vi "art联动采集V4.9(新增双行扫描模块).vi"() -> ()   [LabVIEW 2016]
uses:
  <vilib>/Utility/file.llb/Read Delimited Spreadsheet (I64).vi
  <vilib>/Instr/_visa.llb/VISA Configure Serial Port (Instr).vi
  <vilib>/Utility/file.llb/Write Delimited Spreadsheet (DBL).vi
panel:
  in  "单行？":enum32{"单行", "双行"}(radio)
  in  "色码表导入":path=path "C:/Users/H301/Desktop/art闭环扫描程序/色码表/色码表（黑白）.txt" caption="（色码表导入）"
  out "水平进度条":u8(slide) scale=0.0..100.0
  out "x+y 3":dbl=3.0
  in  "分层图查看":bool
  in  "hDevice 2":i32
  in  "逐行扫描":bool
  in  "定位模式":bool
  in  "X终点":dbl
  in  "Y终点":dbl
  in  "高级设置":bool
  in  "Y轴回零速度":dbl=15000.0
  in  "X轴回零速度":dbl=15000.0
  in  "细分设置":dbl=8.0
  in  "等待时间":u32=40
  in  "文件保存":path=path "C:/Users/H301/Desktop/art采集实验数据" caption="保存路径"
  out "已用时（s）":dbl format="%<%H:%M:%S>t"
  out "error out":errorcluster caption="错误输出"
  in  "退出扫描(Esc)":bool
  in  "N_Length":i32=1048576
  out "M_Length":i32
  out "hDevice":i32=241832032
  out "pulDDR2Length":u32=256
  out "毫秒计时值":u32=3586537
  out "数组":dbl[][](array[numeric])=[[58819.77200735986, 88200.32943600747]]
  out "强度图":dbl[][](graph)=[[58819.77200735986, 88200.32943600747]]
  out "judge":dbl
  out "Xloop":dbl
  out "幅频谱":dbl[](graph)
  out "时域谱":dbl[](graph)
  out "错误输出":errorcluster
  in  "启动":bool
  in  "逐点扫描":bool
  in  "X归零":bool
  in  "Y归零":bool
  in  "Y起点":dbl
  in  "Y轴速度":dbl=9000.0
  in  "X轴速度":dbl=9000.0
  out "电机状态":bool
  in  "电机端口":refnum<visa-resource-name>="COM6"
  out "Yloop":dbl=1.0
  out "X扫描范围":dbl=150.0
  out "Y扫描范围":dbl=75.0
  out "Y序":i32
  in  "X起点":dbl
  out "Y(mm)":dbl
  out "x+y 2":dbl=3.0
  in  "Y:":dbl=1.0
  in  "精度":dbl=0.001
  in  "电机急停":bool
  out "X（mm）":dbl
  out "x+y":dbl=1.0
  in  "X:":dbl=1.0
  # "实时坐标"
  # "时域谱"
  # "频域谱"
  # "归零"
  # "扫描区域"
  # "扫描步进(mm)"
  # "X:"
  # "~"
  # "Y:"
  # "~"
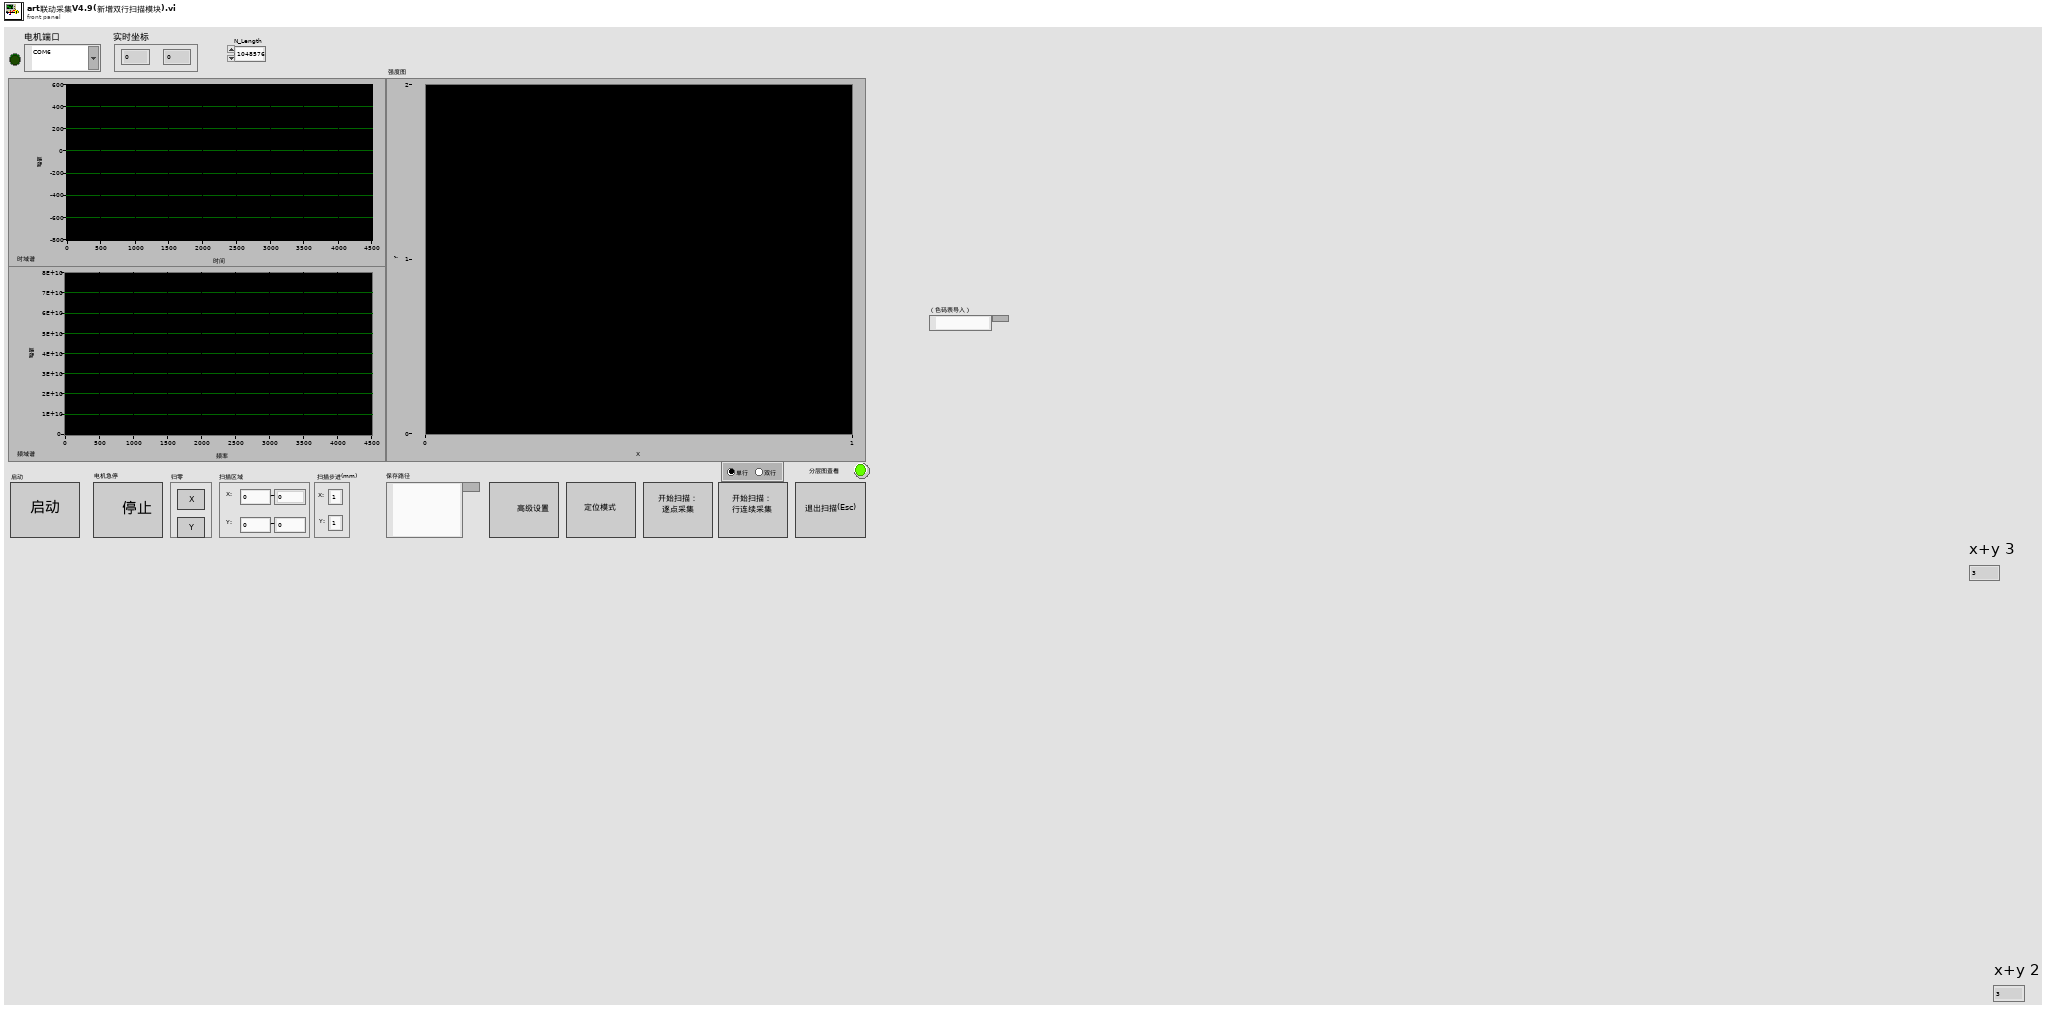
[diagram p1: front panel]
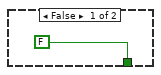
[diagram p2: hidden frame]
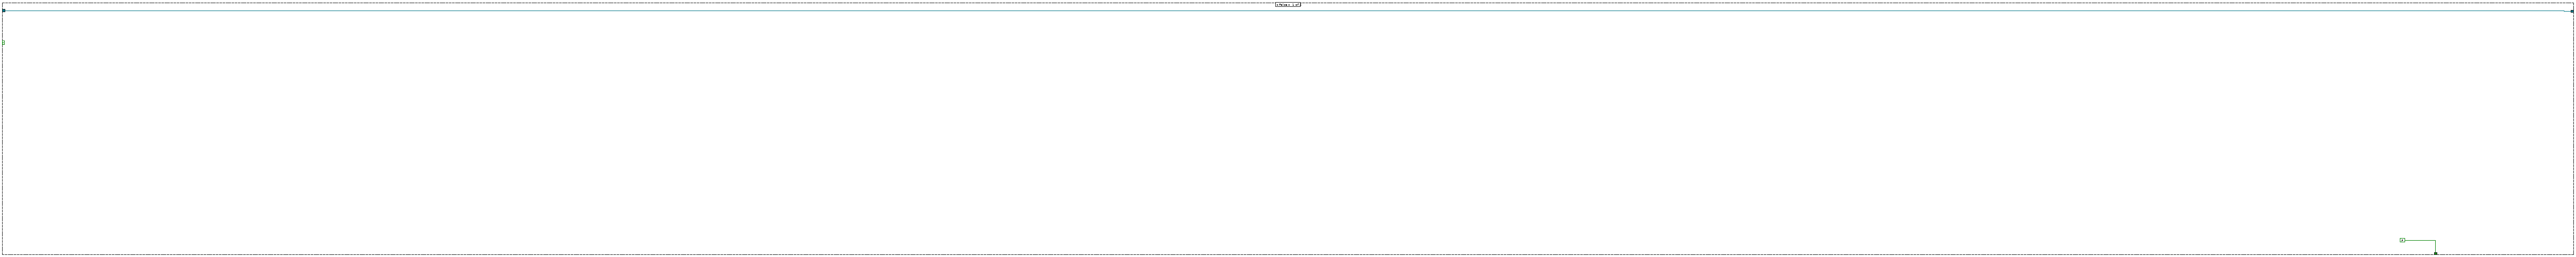
[diagram p3: hidden frame]
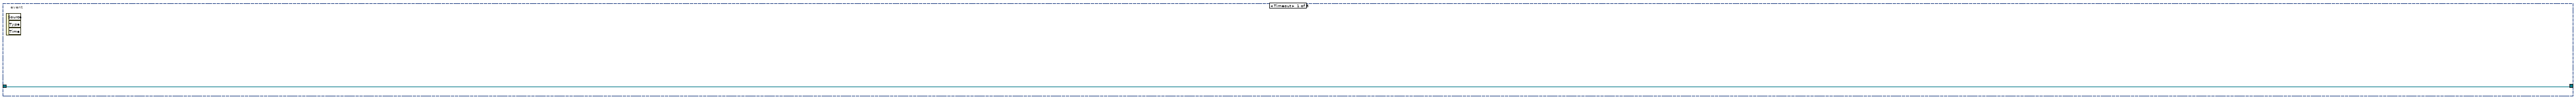
[diagram p4: hidden frame]
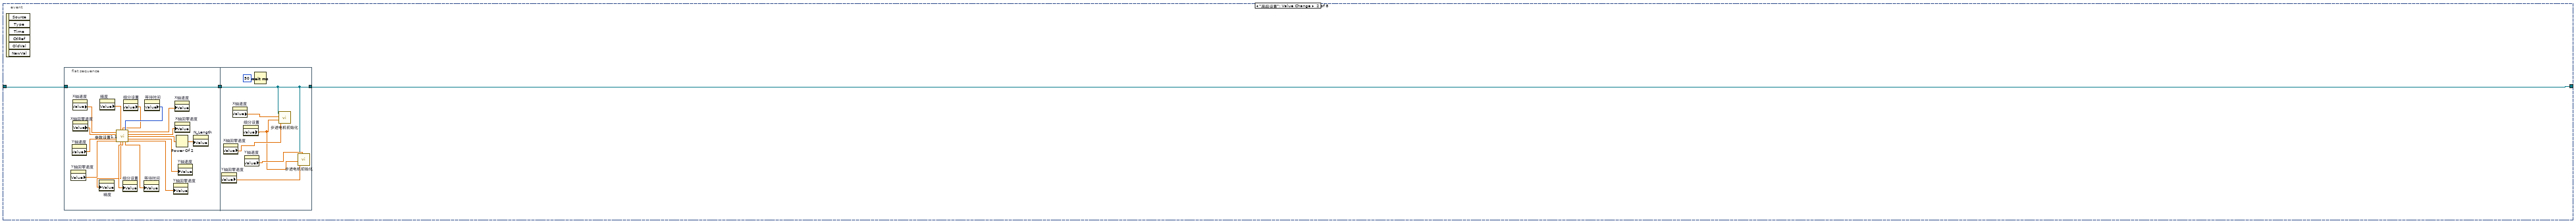
[diagram p5: hidden frame]
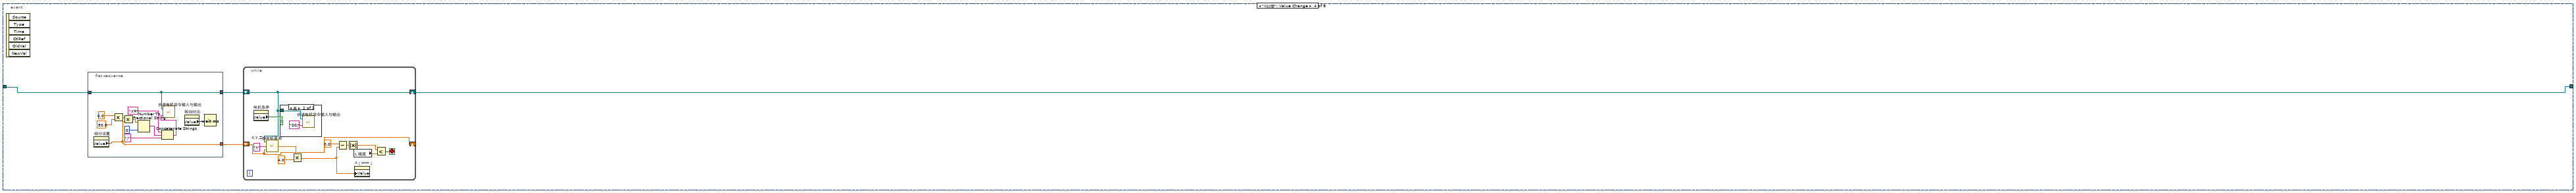
[diagram p6: hidden frame]
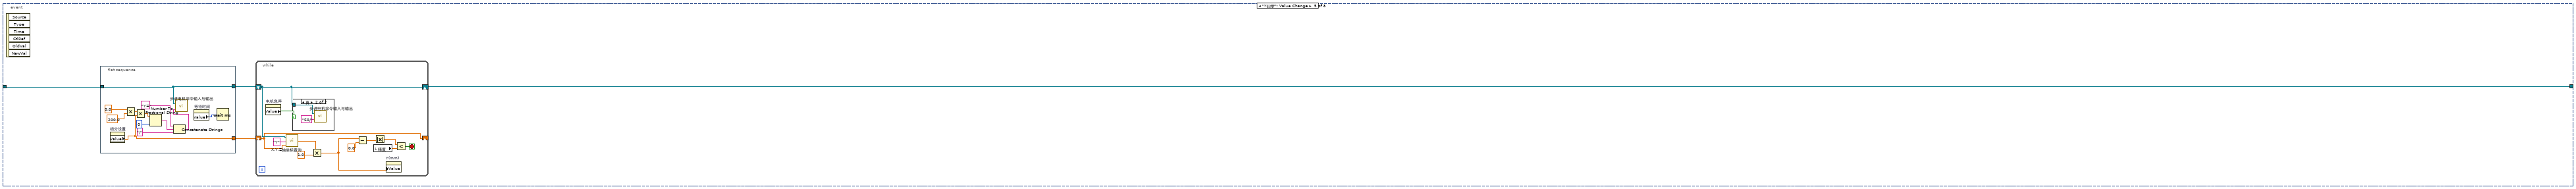
[diagram p8: hidden frame]
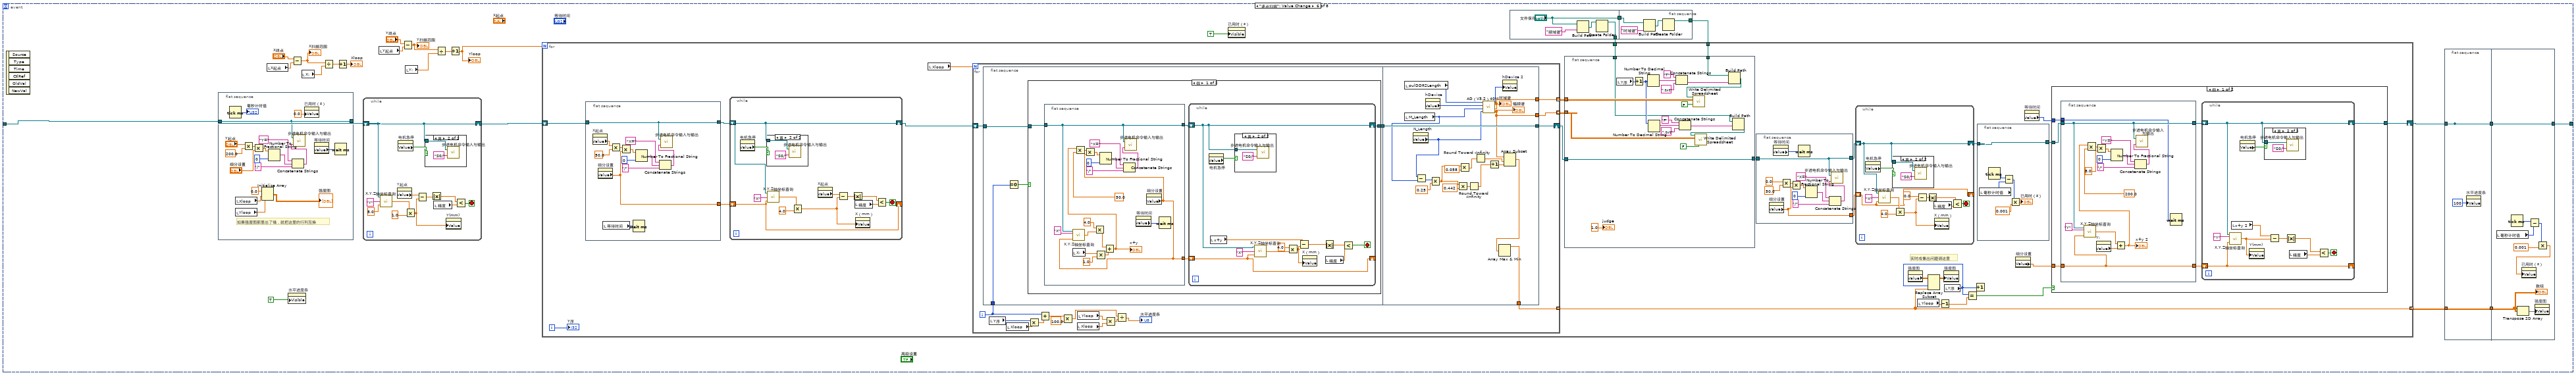
[diagram p10: hidden frame]
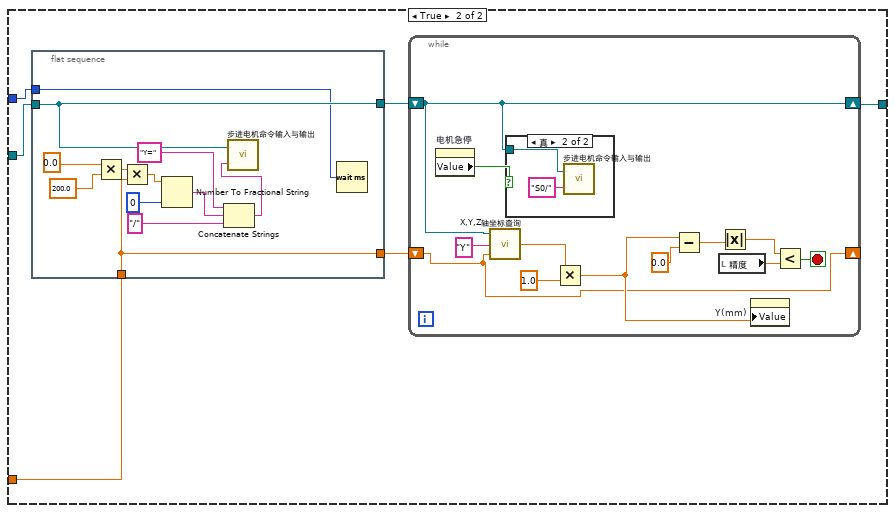
[diagram p15: hidden frame]
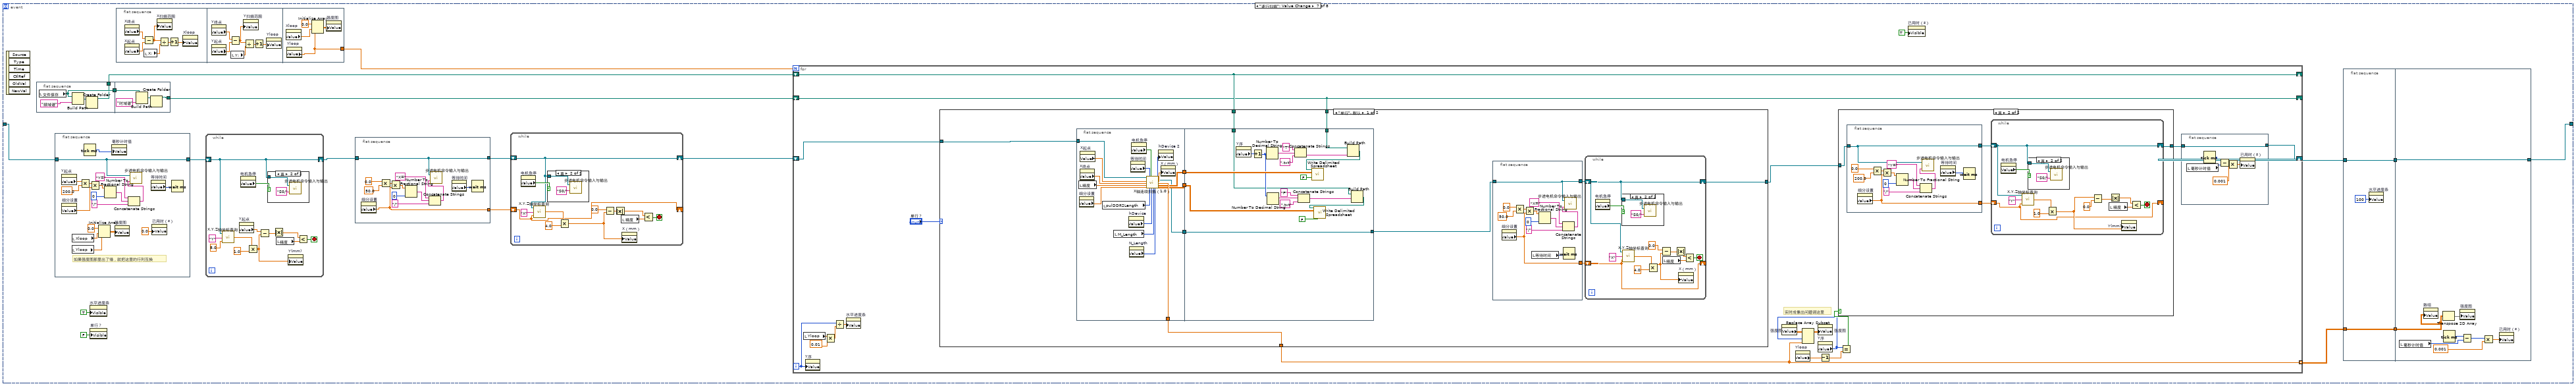
[diagram p19: hidden frame]
diagram:
  n1 = call-poly <vilib>:"Read Delimited Spreadsheet.vi"("file path (dialog if empty)"="色码表导入") -> ("first row"=w2:i64[])  [unwired: 9 in, 5 out]
  n2 = property on="强度图" class="IntGraph (严格)"("Color Table"=w2) -> ()  [unwired: 2 in, 2 out]
  n3 = property on="水平进度条" class="Slide (严格)"("Visible"=FALSE ("可见")) -> ()  [unwired: 2 in, 2 out]
  n4 = property on="单行？" class="RadioBtnsControl (严格)"("Visible"=TRUE ("可见")) -> ()  [unwired: 2 in, 2 out]
  n5 = while {
    stop <- w8 stop-if-true
    n6 = case shown="真" "启动" {
      tunnel: [FALSE ("ESC") w17] -> w8
      frame False {
      }
      frame True {
        w30 = 0  # OutClockSource
        w31 = 0  # bClockSourceDir
        w33 = 40000000  # Frequency
        w34 = 0  # ClockSource
        w35 = 0  # TrigLevelVolt
        w23 = 1
        w36 = 0  # TriggerDir
        w37 = 0  # TriggerSource
        w38 = 0  # ATRTriggerChannel
        w39 = 0  # TriggerMode
        w24 = 0  # M_Length
        w40 = 0  # CouplingType
        w41 = 0  # DeviceLgcID
        w51 = u16 0 items=["无", "XON/XOFF", "RTS/CTS", "XON/XOFF & RTS/CTS", "DTR/DSR", "XON/XOFF & DTR/DSR"] ("flow control (0:none)")
        w52 = u16 10 items=["1.0"=10, "1.5"=15, "2.0"=20] ("stop bits (10: 1 bit)")
        # "3"
        # "2"
        # "1"
        n7 = call-poly "VISA Configure Serial Port"("VISA resource name"="电机端口", "baud rate (9600)"=u32 9600, "data bits (8)"=u16 8, "parity (0:none)"=enum16{"None", "Odd", "Even", "Mark", "Space"}."None", "stop bits (10: 1 bit)"=w52, "flow control (0:none)"=w51) -> ("VISA resource name out"=w43:refnum<visa-resource-name>, "error out"=→"error out":errorcluster)  [unwired: 1 in, 7 out]
        n8 = Build Array "InputRange"(w23, w23, w23, w23) -> (w22:i32[])
        n9 = dll-call lib="PTH2aabs CUsersH301Desktopart闭环扫描程序采集卡控制INFamd64PCI8502_32.dll" fn="PCI8502_CreateDevice" label="CreateDevice"("DeviceLgcID"=w41) -> ("返回类型"=w28:i32)  [unwired: 4 in, 2 out]
        n10 = property on="细分设置" class="DigNum (严格)"() -> ("Value"=w16:dbl)  [unwired: 2 in, 2 out]
        n11 = Build Array (concatenate) "InitDeviceAD"(w33, w22, w40, w24, "N_Length", w39, w38, w37, w36, w35, w34, w31, w30) -> (w32:i32[])
        n12 = call "步进电机初始化.vi"("回零速度"="X轴回零速度", "细分设置"=w16, "X轴速度"="X轴速度", "串口通信端口"=w43) -> ()  [unwired: 2 in, 1 out]
        n13 = dll-call lib="PTH2aabs CUsersH301Desktopart闭环扫描程序采集卡控制INFamd64PCI8502_32.dll" fn="PCI8502_GetDDR2Length" label="GetDDR2Length"("hDevice"=w28, "pulDDR2Length"=u32 0) -> ("hDevice"=w27:i32, "pulDDR2Length"=→"pulDDR2Length":u32)  [unwired: 4 in, 2 out]
        n14 = call "步进电机初始化.vi"("Y轴速度"="Y轴速度", "回零速度"="Y轴回零速度", "细分设置"=w16, "串口通信端口"=w43) -> ()  [unwired: 2 in, 1 out]
        n15 = call "步进电机命令输入与输出.vi"("输入字符串"="?R/", "串口通信端口"=w43) -> ("返回字符串"=w48:string)
        n16 = dll-call lib="PTH2aabs CUsersH301Desktopart闭环扫描程序采集卡控制INFamd64PCI8502_32.dll" fn="PCI8502_InitDeviceAD" label="InitDeviceAD"("hDevice"=w27, "pADPara"=w32) -> ("hDevice"=→"hDevice":i32)  [unwired: 5 in, 2 out]
        n17 = String Subset(string=w48, offset (0)=0 ("偏移量(0)"), length (rest)=2 ("长度（剩余）")) -> (substring=w45:string)
        n18 = Equal?(x=w45, y="OK") -> (x = y?=w42:bool)
        "电机状态" <- w42
        n19 = case shown="真" w42 {
          tunnel: w43 -> [w58 w61]
          tunnel: [w58 w59] -> w18
          tunnel: [FALSE ("ESC") w60] -> w17
          frame False {
          }
          frame True {
            n20 = while {
              tunnel: ["退出扫描(Esc)"] -> w60
              shift-right: [w65] -> w59
              shift-left: w61 -> [w70]
              stop <- "退出扫描(Esc)" stop-if-true
              n21 = property on="水平进度条" class="Slide (严格)"("Visible"=FALSE ("可见")) -> ()  [unwired: 2 in, 2 out]
              n22 = property on="高级设置" class="Bool"("Visible"=TRUE ("可见")) -> ()  [unwired: 2 in, 2 out]
              n23 = property on="定位模式" class="Bool"("Visible"=TRUE ("可见")) -> ()  [unwired: 2 in, 2 out]
              n24 = property on="水平进度条" class="Slide (严格)"("Value"=u8 0 ("水平进度条")) -> ()  [unwired: 2 in, 2 out]
              n25 = property on="单行？" class="RadioBtnsControl (严格)"("Visible"=TRUE ("可见")) -> ()  [unwired: 2 in, 2 out]
              n26 = event shown="[2] \"定位模式\": 值改变" {
                selector: _ -> [_ _ _ _ _ _ _ _]
                dyn-events: _ -> [_ _ _ _ _ _ _ _]
                timeout: 1 -> [_ _ _ _ _ _ _ _]
                tunnel: w70 -> [w71 w74 w107 w111 w141 w192 w506 w871]
                tunnel: [w71 w73 w106 w109 w139 w187 w508 w870] -> w65
                event Timeout {
                  n27 = event-data() -> ()  [unwired: 1 in, 3 out]
                }
                event "高级设置": Value Change {
                  n28 = event-data() -> ()  [unwired: 1 in, 6 out]
                  n29 = flat-sequence {
                    tunnel: w74 -> [w77]
                    tunnel: [w77] -> w72
                    tunnel: [w93] -> w73
                    tunnel: w72 -> [w93]
                    frame #0 {
                      n30 = property on="Y轴回零速度" class="DigNum (严格)"() -> ("Value"=w81:dbl)  [unwired: 2 in, 2 out]
                      n31 = property on="Y轴速度" class="DigNum (严格)"() -> ("Value"=w80:dbl)  [unwired: 2 in, 2 out]
                      n32 = property on="X轴速度" class="DigNum (严格)"() -> ("Value"=w78:dbl)  [unwired: 2 in, 2 out]
                      n33 = property on="X轴回零速度" class="DigNum (严格)"() -> ("Value"=w79:dbl)  [unwired: 2 in, 2 out]
                      n34 = property on="精度" class="DigNum (严格)"() -> ("Value"=w85:dbl)  [unwired: 2 in, 2 out]
                      n35 = property on="细分设置" class="DigNum (严格)"() -> ("Value"=w86:dbl)  [unwired: 2 in, 2 out]
                      n36 = property on="等待时间" class="DigNum (严格)"() -> ("Value"=w87:u32)  [unwired: 2 in, 2 out]
                      n37 = call "参数设置1.1.vi"("X轴速度"=w78, "精度"=w85, "细分设置"=w86, "等待时间"=w87, "X轴回零速度"=w79, "Y轴速度"=w80, "Y轴回零速度"=w81) -> ("X轴速度"=w88:dbl, "X轴回零速度"=w89:dbl, "采样阶"=w75:dbl, "Y轴速度"=w90:dbl, "精度"=w82:dbl, "细分设置"=w83:dbl, "等待时间"=w84:dbl, "Y轴回零速度"=w91:dbl)  [unwired: 1 in]
                      n38 = property on="精度" class="DigNum (严格)"("Value"=w82) -> ()  [unwired: 2 in, 2 out]
                      n39 = property on="细分设置" class="DigNum (严格)"("Value"=w83) -> ()  [unwired: 2 in, 2 out]
                      n40 = property on="等待时间" class="DigNum (严格)"("Value"=w84) -> ()  [unwired: 2 in, 2 out]
                      n41 = property on="Y轴回零速度" class="DigNum (严格)"("Value"=w91) -> ()  [unwired: 2 in, 2 out]
                      n42 = property on="X轴速度" class="DigNum (严格)"("Value"=w88) -> ()  [unwired: 2 in, 2 out]
                      n43 = property on="X轴回零速度" class="DigNum (严格)"("Value"=w89) -> ()  [unwired: 2 in, 2 out]
                      n44 = Power Of 2(x=w75) -> (2^x=w76:dbl)
                      n45 = property on="Y轴速度" class="DigNum (严格)"("Value"=w90) -> ()  [unwired: 2 in, 2 out]
                      n46 = property on="N_Length" class="DigNum (严格)"("Value"=w76) -> ()  [unwired: 2 in, 2 out]
                    }
                    frame #1 {
                      n47 = property on="Y轴回零速度" class="DigNum (严格)"() -> ("Value"=w97:dbl)  [unwired: 2 in, 2 out]
                      n48 = property on="X轴回零速度" class="DigNum (严格)"() -> ("Value"=w96:dbl)  [unwired: 2 in, 2 out]
                      n49 = property on="X轴速度" class="DigNum (严格)"() -> ("Value"=w95:dbl)  [unwired: 2 in, 2 out]
                      n50 = property on="细分设置" class="DigNum (严格)"() -> ("Value"=w94:dbl)  [unwired: 2 in, 2 out]
                      n51 = property on="Y轴速度" class="DigNum (严格)"() -> ("Value"=w98:dbl)  [unwired: 2 in, 2 out]
                      n52 = Wait (ms)(milliseconds to wait=u32 50 ("等待时间（毫秒）")) -> ()  [unwired: 1 out]
                      n53 = call "步进电机初始化.vi"("回零速度"=w96, "细分设置"=w94, "X轴速度"=w95, "串口通信端口"=w93) -> ()  [unwired: 2 in, 1 out]
                      n54 = call "步进电机初始化.vi"("Y轴速度"=w98, "回零速度"=w97, "细分设置"=w94, "串口通信端口"=w93) -> ()  [unwired: 2 in, 1 out]
                    }
                  }
                }
                event "定位模式": Value Change {
                  n55 = event-data() -> ()  [unwired: 1 in, 6 out]
                  n56 = local read "pulDDR2Length"() -> (w103:u32)
                  n57 = local read "M_Length"() -> (w101:i32)
                  n58 = property on="hDevice" class="DigNum (严格)"() -> ("Value"=w102:i32)  [unwired: 2 in, 2 out]
                  n59 = property on="N_Length" class="DigNum (严格)"() -> ("Value"=w100:i32)  [unwired: 2 in, 2 out]
                  n60 = call "电机定位1.1（40M只处理采集卡）.vi"("VISA I"=w107, "pulDDR2Length"=w103, "hDevice"=w102, "M-length"=w101, "N-length"=w100) -> ("hDevice out"=w99:i32, "VISA O"=w106:refnum<visa-resource-name>, "X"=w105:dbl, "Y"=w104:dbl)  [unwired: 11 in]
                  n61 = property on="hDevice 2" class="DigNum (严格)"("Value"=w99) -> ()  [unwired: 2 in, 2 out]
                  n62 = property on="X（mm）" class="DigNum (严格)"("Value"=w105) -> ()  [unwired: 2 in, 2 out]
                  n63 = property on="Y(mm)" class="DigNum (严格)"("Value"=w104) -> ()  [unwired: 2 in, 2 out]
                }
                event "X归零": Value Change {
                  n64 = event-data() -> ()  [unwired: 1 in, 6 out]
                  n65 = flat-sequence {
                    tunnel: w111 -> [w115]
                    tunnel: [w115] -> w110
                    tunnel: [w112] -> w108
                    frame #0 {
                      n66 = property on="细分设置" class="DigNum (严格)"() -> ("Value"=w112:dbl)  [unwired: 2 in, 2 out]
                      n67 = Multiply(x=0.0, y=50.0) -> (x*y=w118:dbl)
                      n68 = Multiply(x=w118, y=w112) -> (x*y=w123:dbl)
                      n69 = Number To Fractional String(number=w123, precision (6)=i16 0 ("精度(6)")) -> (F-format string=w121:string)  [unwired: 2 out]
                      n70 = Concatenate Strings("X=" ("字符串"), w121, "/" ("字符串")) -> (w116:string)
                      n71 = call "步进电机命令输入与输出.vi"("输入字符串"=w116, "串口通信端口"=w115) -> ()  [unwired: 1 out]
                      n72 = property on="等待时间" class="DigNum (严格)"() -> ("Value"=w113:u32)  [unwired: 2 in, 2 out]
                      n73 = Wait (ms)(milliseconds to wait=w113) -> ()  [unwired: 1 out]
                    }
                  }
                  n74 = while {
                    shift-right: [w125] -> w109
                    shift-left: w110 -> [w125]
                    shift-right: [w124] -> _
                    shift-left: w108 -> [w124]
                    stop <- w131 stop-if-true
                    n75 = property on="电机急停" class="Bool (严格)"() -> ("Value"=w132:bool)  [unwired: 2 in, 2 out]
                    n76 = call "X,Y,Z轴坐标查询.vi"("细分设置"=w124, "查询坐标轴"="X", "串口通信端口"=w125) -> ("坐标(mm)"=w133:dbl)
                    n77 = case shown="真" w132 {
                      tunnel: w125 -> [_ w136]
                      frame False {
                      }
                      frame True {
                        n78 = call "步进电机命令输入与输出.vi"("输入字符串"="S0/", "串口通信端口"=w136) -> ()  [unwired: 1 out]
                      }
                    }
                    n79 = Multiply(x=w133, y=4.0 ("x")) -> (x*y=w129:dbl)
                    n80 = Subtract(x=0.0, y=w129) -> (x-y=w128:dbl)
                    n81 = Absolute Value(x=w128) -> (abs(x)=w127:dbl)
                    n82 = local read "精度"() -> (w130:dbl)
                    n83 = property on="X（mm）" class="DigNum (严格)"("Value"=w129) -> ()  [unwired: 2 in, 2 out]
                    n84 = Less?(x=w127, y=w130) -> (x < y?=w131:bool)
                  }
                }
                event "Y归零": Value Change {
                  n85 = event-data() -> ()  [unwired: 1 in, 6 out]
                  n86 = flat-sequence {
                    tunnel: w141 -> [w145]
                    tunnel: [w145] -> w140
                    tunnel: [w142] -> w138
                    frame #0 {
                      n87 = property on="细分设置" class="DigNum (严格)"() -> ("Value"=w142:dbl)  [unwired: 2 in, 2 out]
                      n88 = Multiply(x=0.0, y=200.0) -> (x*y=w148:dbl)
                      n89 = Multiply(x=w148, y=w142) -> (x*y=w153:dbl)
                      n90 = Number To Fractional String(number=w153, precision (6)=i16 0 ("精度(6)")) -> (F-format string=w151:string)  [unwired: 2 out]
                      n91 = Concatenate Strings("Y=" ("字符串"), w151, "/" ("字符串")) -> (w146:string)
                      n92 = call "步进电机命令输入与输出.vi"("输入字符串"=w146, "串口通信端口"=w145) -> ()  [unwired: 1 out]
                      n93 = property on="等待时间" class="DigNum (严格)"() -> ("Value"=w143:u32)  [unwired: 2 in, 2 out]
                      n94 = Wait (ms)(milliseconds to wait=w143) -> ()  [unwired: 1 out]
                    }
                  }
                  n95 = while {
                    shift-right: [w155] -> w139
                    shift-left: w140 -> [w155]
                    shift-right: [w154] -> _
                    shift-left: w138 -> [w154]
                    stop <- w161 stop-if-true
                    n96 = property on="电机急停" class="Bool (严格)"() -> ("Value"=w162:bool)  [unwired: 2 in, 2 out]
                    n97 = call "X,Y,Z轴坐标查询.vi"("细分设置"=w154, "查询坐标轴"="Y", "串口通信端口"=w155) -> ("坐标(mm)"=w163:dbl)
                    n98 = case shown="真" w162 {
                      tunnel: w155 -> [_ w166]
                      frame False {
                      }
                      frame True {
                        n99 = call "步进电机命令输入与输出.vi"("输入字符串"="S0/", "串口通信端口"=w166) -> ()  [unwired: 1 out]
                      }
                    }
                    n100 = Multiply(x=w163, y=1.0 ("x")) -> (x*y=w159:dbl)
                    n101 = Subtract(x=w159, y=0.0 ("x")) -> (x-y=w157:dbl)
                    n102 = local read "精度"() -> (w160:dbl)
                    n103 = Absolute Value(x=w157) -> (abs(x)=w156:dbl)
                    n104 = property on="Y(mm)" class="DigNum (严格)"("Value"=w159) -> ()  [unwired: 2 in, 2 out]
                    n105 = Less?(x=w156, y=w160) -> (x < y?=w161:bool)
                  }
                }
                event "逐点扫描": Value Change {
                  n106 = event-data() -> ()  [unwired: 1 in, 6 out]
                  n107 = flat-sequence {
                    tunnel: w192 -> [w221]
                    tunnel: [w221] -> w183
                    frame #0 {
                      # "如果强度图那里出了错，就把这里的行列互换"
                      n108 = Tick Count (ms)() -> (millisecond timer value=→"毫秒计时值":u32)
                      n109 = local read "Xloop"() -> (w216:dbl)
                      n110 = local read "Yloop"() -> (w215:dbl)
                      n111 = Multiply(x="Y起点", y=200.0) -> (x*y=w224:dbl)
                      n112 = Multiply(x=w224, y="细分设置") -> (x*y=w229:dbl)
                      n113 = Initialize Array(0.0 ("元素"), w216, w215) -> (→"强度图":dbl[][])
                      n114 = Number To Fractional String(number=w229, precision (6)=i16 0 ("精度(6)")) -> (F-format string=w227:string)  [unwired: 2 out]
                      n115 = Concatenate Strings("Y=" ("字符串"), w227, "/" ("字符串")) -> (w222:string)
                      n116 = call "步进电机命令输入与输出.vi"("输入字符串"=w222, "串口通信端口"=w221) -> ()  [unwired: 1 out]
                      n117 = property on="已用时（s）" class="DigNum (严格)"("Value"=0.0 ("已用时（s）")) -> ()  [unwired: 2 in, 2 out]
                      n118 = property on="等待时间" class="DigNum (严格)"() -> ("Value"=w213:u32)  [unwired: 2 in, 2 out]
                      n119 = Wait (ms)(milliseconds to wait=w213) -> ()  [unwired: 1 out]
                    }
                  }
                  n120 = local read "X起点"() -> (w179:dbl)
                  n121 = property on="水平进度条" class="Slide (严格)"("Visible"=TRUE ("可见")) -> ()  [unwired: 2 in, 2 out]
                  n122 = Subtract(x="X终点", y=w179) -> (x-y=w178:dbl)
                  "X扫描范围" <- w178
                  n123 = local read "X:"() -> (w186:dbl)
                  n124 = Divide(x=w178, y=w186) -> (x/y=w184:dbl)
                  n125 = Increment(x=w184) -> (x+1=→"Xloop":dbl)
                  n126 = while {
                    shift-right: [w230] -> w175
                    shift-left: w183 -> [w230]
                    stop <- w235 stop-if-true
                    n127 = call "X,Y,Z轴坐标查询.vi"("细分设置"=8.0, "查询坐标轴"="Y", "串口通信端口"=w230) -> ("坐标(mm)"=w237:dbl)
                    n128 = property on="Y起点" class="DigNum (严格)"() -> ("Value"=w239:dbl)  [unwired: 2 in, 2 out]
                    n129 = property on="电机急停" class="Bool (严格)"() -> ("Value"=w236:bool)  [unwired: 2 in, 2 out]
                    n130 = Multiply(x=w237, y=1.0 ("x")) -> (x*y=w233:dbl)
                    n131 = Subtract(x=w239, y=w233) -> (x-y=w232:dbl)
                    n132 = case shown="真" w236 {
                      tunnel: w230 -> [_ w242]
                      frame False {
                      }
                      frame True {
                        n133 = call "步进电机命令输入与输出.vi"("输入字符串"="S0/", "串口通信端口"=w242) -> ()  [unwired: 1 out]
                      }
                    }
                    n134 = Absolute Value(x=w232) -> (abs(x)=w231:dbl)
                    n135 = local read "精度"() -> (w234:dbl)
                    n136 = property on="Y(mm)" class="DigNum (严格)"("Value"=w233) -> ()  [unwired: 2 in, 2 out]
                    n137 = Less?(x=w231, y=w234) -> (x < y?=w235:bool)
                  }
                  n138 = local read "Y起点"() -> (w181:dbl)
                  n139 = Subtract(x="Y终点", y=w181) -> (x-y=w177:dbl)
                  "Y扫描范围" <- w177
                  n140 = local read "Y:"() -> (w191:dbl)
                  n141 = Divide(x=w177, y=w191) -> (x/y=w190:dbl)
                  n142 = Increment(x=w190) -> (x+1=w189:dbl)
                  "Yloop" <- w189
                  n143 = for {
                    N: w189 -> [_]
                    shift-right: [w267] -> w168
                    shift-left: w175 -> [w248]
                    tunnel: [w250] -> w188 mode=indexing
                    tunnel: w173 -> [w254]
                    tunnel: w176 -> [w253]
                    i -> [w268]
                    # "实时成像出问题调这里"
                    n144 = flat-sequence {
                      tunnel: w248 -> [w325]
                      tunnel: [w325] -> w266
                      tunnel: [w324] -> w258
                      frame #0 {
                        n145 = property on="X起点" class="DigNum (严格)"() -> ("Value"=w322:dbl)  [unwired: 2 in, 2 out]
                        n146 = property on="细分设置" class="DigNum (严格)"() -> ("Value"=w324:dbl)  [unwired: 2 in, 2 out]
                        n147 = local read "等待时间"() -> (w323:u32)
                        n148 = Multiply(x=w322, y=50.0) -> (x*y=w328:dbl)
                        n149 = Multiply(x=w328, y=w324) -> (x*y=w333:dbl)
                        n150 = Wait (ms)(milliseconds to wait=w323) -> ()  [unwired: 1 out]
                        n151 = Number To Fractional String(number=w333, precision (6)=i16 0 ("精度(6)")) -> (F-format string=w331:string)  [unwired: 2 out]
                        n152 = Concatenate Strings("X=" ("字符串"), w331, "/" ("字符串")) -> (w326:string)
                        n153 = call "步进电机命令输入与输出.vi"("输入字符串"=w326, "串口通信端口"=w325) -> ()  [unwired: 1 out]
                      }
                    }
                    n154 = while {
                      shift-right: [w335] -> w246
                      shift-left: w266 -> [w335]
                      shift-right: [w334] -> _
                      shift-left: w258 -> [w334]
                      stop <- w340 stop-if-true
                      n155 = property on="电机急停" class="Bool (严格)"() -> ("Value"=w341:bool)  [unwired: 2 in, 2 out]
                      n156 = case shown="真" w341 {
                        tunnel: w335 -> [_ w346]
                        frame False {
                        }
                        frame True {
                          n157 = call "步进电机命令输入与输出.vi"("输入字符串"="S0/", "串口通信端口"=w346) -> ()  [unwired: 1 out]
                        }
                      }
                      n158 = call "X,Y,Z轴坐标查询.vi"("细分设置"=w334, "查询坐标轴"="X", "串口通信端口"=w335) -> ("坐标(mm)"=w342:dbl)
                      n159 = Multiply(x=w342, y=4.0 ("x")) -> (x*y=w338:dbl)
                      n160 = property on="X起点" class="DigNum (严格)"() -> ("Value"=w344:dbl)  [unwired: 2 in, 2 out]
                      n161 = Subtract(x=w344, y=w338) -> (x-y=w337:dbl)
                      n162 = Absolute Value(x=w337) -> (abs(x)=w336:dbl)
                      n163 = local read "精度"() -> (w339:dbl)
                      n164 = property on="X（mm）" class="DigNum (严格)"("Value"=w338) -> ()  [unwired: 2 in, 2 out]
                      n165 = Less?(x=w336, y=w339) -> (x < y?=w340:bool)
                    }
                    n166 = local read "Xloop"() -> (w259:dbl)
                    n167 = for {
                      N: w259 -> [_]
                      shift-right: [w429] -> w247
                      shift-left: w246 -> [w425]
                      tunnel: [w428] -> w265 mode=indexing
                      tunnel: [w427] -> w264 mode=indexing
                      tunnel: [w426] -> w250 mode=indexing
                      i -> [w417]
                      n168 = flat-sequence {
                        tunnel: w425 -> [w434]
                        tunnel: [w433] -> w430
                        tunnel: w417 -> [w431]
                        tunnel: [w492] -> w429
                        tunnel: w430 -> [w492]
                        tunnel: [w491] -> w428
                        tunnel: [w490] -> w427
                        tunnel: [w488] -> w426
                        frame #0 {
                          n169 = Equal To 0?(x=w431) -> (x = 0?=w432:bool)
                          n170 = case shown="假" w432 {
                            tunnel: w434 -> [w437 w472]
                            tunnel: [w436 w472] -> w433
                            frame False {
                              n171 = flat-sequence {
                                tunnel: w437 -> [w447]
                                tunnel: [w447] -> w438
                                tunnel: [w439] -> w435
                                frame #0 {
                                n172 = local read "X:"() -> (w441:dbl)
                                n173 = Multiply(x=w441, y=1.0 ("x")) -> (x*y=w446:dbl)
                                n174 = property on="等待时间" class="DigNum (严格)"() -> ("Value"=w440:u32)  [unwired: 2 in, 2 out]
                                n175 = property on="细分设置" class="DigNum (严格)"() -> ("Value"=w439:dbl)  [unwired: 2 in, 2 out]
                                n176 = call "X,Y,Z轴坐标查询.vi"("细分设置"=w439, "查询坐标轴"="X", "串口通信端口"=w447) -> ("坐标(mm)"=w443:dbl)
                                n177 = Multiply(x=4.0, y=w443) -> (x*y=w442:dbl)
                                n178 = Add(x=w442, y=w446) -> (x+y=w449:dbl)
                                "x+y" <- w449
                                n179 = Multiply(x=w449, y=50.0) -> (x*y=w452:dbl)
                                n180 = Multiply(x=w452, y=w439) -> (x*y=w457:dbl)
                                n181 = Number To Fractional String(number=w457, precision (6)=i16 0 ("精度(6)")) -> (F-format string=w455:string)  [unwired: 2 out]
                                n182 = Concatenate Strings("X=" ("字符串"), w455, "/" ("字符串")) -> (w450:string)
                                n183 = call "步进电机命令输入与输出.vi"("输入字符串"=w450, "串口通信端口"=w447) -> ()  [unwired: 1 out]
                                n184 = Wait (ms)(milliseconds to wait=w440) -> ()  [unwired: 1 out]
                                }
                              }
                              n185 = while {
                                shift-right: [w467] -> w436
                                shift-left: w438 -> [w467]
                                shift-right: [w458] -> _
                                shift-left: w435 -> [w458]
                                stop <- w466 stop-if-true
                                n186 = property on="电机急停" class="Bool (严格)"() -> ("Value"=w464:bool)  [unwired: 2 in, 2 out]
                                n187 = local read "x+y"() -> (w468:dbl)
                                n188 = case shown="真" w464 {
                                tunnel: w467 -> [_ w470]
                                frame False {
                                }
                                frame True {
                                n189 = call "步进电机命令输入与输出.vi"("输入字符串"="S0/", "串口通信端口"=w470) -> ()  [unwired: 1 out]
                                }
                                }
                                n190 = call "X,Y,Z轴坐标查询.vi"("细分设置"=w458, "查询坐标轴"="X", "串口通信端口"=w467) -> ("坐标(mm)"=w462:dbl)
                                n191 = Multiply(x=4.0, y=w462) -> (x*y=w461:dbl)
                                n192 = Subtract(x=w468, y=w461) -> (x-y=w460:dbl)
                                n193 = property on="X（mm）" class="DigNum (严格)"("Value"=w461) -> ()  [unwired: 2 in, 2 out]
                                n194 = Absolute Value(x=w460) -> (abs(x)=w459:dbl)
                                n195 = local read "精度"() -> (w463:dbl)
                                n196 = Less?(x=w459, y=w463) -> (x < y?=w466:bool)
                              }
                            }
                            frame True {
                            }
                          }
                        }
                        frame #1 {
                          n197 = local read "pulDDR2Length"() -> (w487:u32)
                          n198 = local read "M_Length"() -> (w486:i32)
                          n199 = property on="N_Length" class="DigNum (严格)"() -> ("Value"=w475:i32)  [unwired: 2 in, 2 out]
                          n200 = Subtract(x=w475, y=w486) -> (x-y=w484:i32)
                          n201 = property on="hDevice" class="DigNum (严格)"() -> ("Value"=w473:i32)  [unwired: 2 in, 2 out]
                          n202 = Multiply(x=w484, y=0.25) -> (x*y=w477:dbl)
                          n203 = Multiply(x=w477, y=0.442) -> (x*y=w479:dbl)
                          n204 = Multiply(x=w477, y=0.058) -> (x*y=w481:dbl)
                          n205 = Round Toward -Infinity(1:w479) -> (0:w476:dbl)
                          n206 = Round Toward -Infinity(1:w481) -> (0:w480:dbl)
                          n207 = call "AD（V3.2）40M.vi"("N-length"=w475, "M-length"=w486, "hDevice"=w473, "pulDDR2Length"=w487) -> ("幅频谱"=w490:dbl[], "时域谱"=w491:dbl[], "hDevice out"=w474:i32)  [unwired: 5 in]
                          "时域谱" <- w491
                          "幅频谱" <- w490
                          n208 = Increment(x=w476) -> (x+1=w483:dbl)
                          n209 = property on="hDevice 2" class="DigNum (严格)"("Value"=w474) -> ()  [unwired: 2 in, 2 out]
                          n210 = Array Subset(array=w490, index=w480, length=w483) -> (w489:dbl[])
                          n211 = Array Max & Min(array=w489) -> (max value=w488:dbl)  [unwired: 3 out]
                        }
                      }
                      n212 = local read "Y序"() -> (w419:i32)
                      n213 = local read "Xloop"() -> (w420:dbl)
                      n214 = Multiply(x=w419, y=w420) -> (x*y=w418:dbl)
                      n215 = Add(x=w417, y=w418) -> (x+y=w416:dbl)
                      n216 = Multiply(x=w416, y=100.0) -> (x*y=w414:dbl)
                      n217 = local read "Xloop"() -> (w424:dbl)
                      n218 = local read "Yloop"() -> (w423:dbl)
                      n219 = Multiply(x=w423, y=w424) -> (x*y=w422:dbl)
                      n220 = Divide(x=w414, y=w422) -> (x/y=→"水平进度条":dbl)
                    }
                    n221 = flat-sequence {
                      tunnel: w264 -> [w308]
                      tunnel: w265 -> [w316]
                      tunnel: w247 -> [w320]
                      tunnel: [w320] -> w260
                      tunnel: w254 -> [w303]
                      tunnel: w253 -> [w302]
                      frame #0 {
                        n222 = local read "Y序"() -> (w304:i32)
                        n223 = Increment(x=w304) -> (x+1=w305:i32)
                        n224 = Number To Decimal String(number=w305) -> (decimal integer string=w314:string)  [unwired: 1 in]
                        n225 = Number To Decimal String(number=w305) -> (decimal integer string=w313:string)  [unwired: 1 in]
                        n226 = Concatenate Strings("T" ("字符串"), w314, ".txt" ("字符串")) -> (w317:string)
                        n227 = Concatenate Strings("F" ("字符串"), w313, ".txt" ("字符串")) -> (w311:string)
                        n228 = Build Path(base path=w303, name or relative path=w317) -> (appended path=w319:path)
                        n229 = call-poly <vilib>:"Write Delimited Spreadsheet.vi"("file path (dialog if empty)"=w319, "2D data"=w316, "transpose? (no:F)"=FALSE) -> ()  [unwired: 11 in, 2 out]
                        n230 = Build Path(base path=w302, name or relative path=w311) -> (appended path=w309:path)
                        n231 = call-poly <vilib>:"Write Delimited Spreadsheet.vi"("file path (dialog if empty)"=w309, "2D data"=w308, "transpose? (no:F)"=FALSE) -> ()  [unwired: 11 in, 2 out]
                        "judge" <- 1.0
                      }
                    }
                    n232 = flat-sequence {
                      tunnel: w260 -> [w279]
                      tunnel: [w279] -> w261
                      tunnel: [w277] -> w257
                      frame #0 {
                        n233 = property on="细分设置" class="DigNum (严格)"() -> ("Value"=w277:dbl)  [unwired: 2 in, 2 out]
                        n234 = property on="等待时间" class="DigNum (严格)"() -> ("Value"=w276:u32)  [unwired: 2 in, 2 out]
                        n235 = Multiply(x=0.0, y=50.0) -> (x*y=w282:dbl)
                        n236 = Multiply(x=w282, y=w277) -> (x*y=w287:dbl)
                        n237 = Wait (ms)(milliseconds to wait=w276) -> ()  [unwired: 1 out]
                        n238 = Number To Fractional String(number=w287, precision (6)=i16 0 ("精度(6)")) -> (F-format string=w285:string)  [unwired: 2 out]
                        n239 = Concatenate Strings("X=" ("字符串"), w285, "/" ("字符串")) -> (w280:string)
                        n240 = call "步进电机命令输入与输出.vi"("输入字符串"=w280, "串口通信端口"=w279) -> ()  [unwired: 1 out]
                      }
                    }
                    n241 = while {
                      shift-right: [w289] -> w245
                      shift-left: w261 -> [w289]
                      shift-right: [w288] -> _
                      shift-left: w257 -> [w288]
                      stop <- w295 stop-if-true
                      n242 = property on="电机急停" class="Bool (严格)"() -> ("Value"=w296:bool)  [unwired: 2 in, 2 out]
                      n243 = call "X,Y,Z轴坐标查询.vi"("细分设置"=w288, "查询坐标轴"="X", "串口通信端口"=w289) -> ("坐标(mm)"=w297:dbl)
                      n244 = case shown="真" w296 {
                        tunnel: w289 -> [_ w300]
                        frame False {
                        }
                        frame True {
                          n245 = call "步进电机命令输入与输出.vi"("输入字符串"="S0/", "串口通信端口"=w300) -> ()  [unwired: 1 out]
                        }
                      }
                      n246 = Multiply(x=w297, y=4.0 ("x")) -> (x*y=w293:dbl)
                      n247 = Subtract(x=0.0, y=w293) -> (x-y=w292:dbl)
                      n248 = Absolute Value(x=w292) -> (abs(x)=w291:dbl)
                      n249 = local read "精度"() -> (w294:dbl)
                      n250 = property on="X（mm）" class="DigNum (严格)"("Value"=w293) -> ()  [unwired: 2 in, 2 out]
                      n251 = Less?(x=w291, y=w294) -> (x < y?=w295:bool)
                    }
                    n252 = property on="强度图" class="IntGraph (严格)"() -> ("Value"=w251:dbl[][])  [unwired: 2 in, 2 out]
                    n253 = local read "Yloop"() -> (w262:dbl)
                    n254 = Decrement(x=w262) -> (x-1=w263:dbl)
                    n255 = local read "Y序"() -> (w249:i32)
                    n256 = Replace Array Subset(array=w251, new element=w250, index (col)=w249) -> (w252:dbl[][])  [unwired: 1 in]
                    n257 = property on="强度图" class="IntGraph (严格)"("Value"=w252) -> ()  [unwired: 2 in, 2 out]
                    n258 = Equal?(x=w249, y=w263) -> (x = y?=w269:bool)
                    n259 = Increment(x=w249) -> ()  [unwired: 1 out]
                    n260 = flat-sequence {
                      tunnel: w245 -> [w275]
                      tunnel: [w275] -> w244
                      frame #0 {
                        n261 = local read "毫秒计时值"() -> (w270:u32)
                        n262 = Tick Count (ms)() -> (millisecond timer value=w274:u32)
                        n263 = Subtract(x=w274, y=w270) -> (x-y=w271:u32)
                        n264 = Multiply(x=w271, y=0.001) -> (x*y=→"已用时（s）":dbl)
                      }
                    }
                    n265 = property on="细分设置" class="DigNum (严格)"() -> ("Value"=w255:dbl)  [unwired: 2 in, 2 out]
                    n266 = property on="等待时间" class="DigNum (严格)"() -> ("Value"=w256:u32)  [unwired: 2 in, 2 out]
                    n267 = case shown="假" w269 {
                      tunnel: w244 -> [w353 w385]
                      tunnel: [w351 w386] -> w267
                      tunnel: w256 -> [w349 w383]
                      tunnel: w255 -> [w348 w382]
                      frame False {
                        n268 = flat-sequence {
                          tunnel: w353 -> [w357]
                          tunnel: [w357] -> w352
                          tunnel: [w355] -> w350
                          tunnel: w349 -> [w356]
                          tunnel: w348 -> [w355]
                          frame #0 {
                            n269 = call "X,Y,Z轴坐标查询.vi"("细分设置"=w355, "查询坐标轴"="Y", "串口通信端口"=w357) -> ("坐标(mm)"=w358:dbl)
                            n270 = property on="Y:" class="DigNum (严格)"() -> ("Value"=w354:dbl)  [unwired: 2 in, 2 out]
                            n271 = Add(x=w358, y=w354) -> (x+y=w360:dbl)
                            "x+y 2" <- w360
                            n272 = Multiply(x=w360, y=200.0) -> (x*y=w364:dbl)
                            n273 = Multiply(x=w364, y=8.0 ("细分设置")) -> (x*y=w369:dbl)
                            n274 = Number To Fractional String(number=w369, precision (6)=i16 0 ("精度(6)")) -> (F-format string=w367:string)  [unwired: 2 out]
                            n275 = Concatenate Strings("Y=" ("字符串"), w367, "/" ("字符串")) -> (w362:string)
                            n276 = call "步进电机命令输入与输出.vi"("输入字符串"=w362, "串口通信端口"=w357) -> ()  [unwired: 1 out]
                            n277 = Wait (ms)(milliseconds to wait=w356) -> ()  [unwired: 1 out]
                          }
                        }
                        n278 = while {
                          shift-right: [w371] -> w351
                          shift-left: w352 -> [w371]
                          shift-right: [w370] -> _
                          shift-left: w350 -> [w370]
                          stop <- w377 stop-if-true
                          n279 = call "X,Y,Z轴坐标查询.vi"("细分设置"=w370, "查询坐标轴"="Y", "串口通信端口"=w371) -> ("坐标(mm)"=w375:dbl)
                          n280 = local read "x+y 2"() -> (w378:dbl)
                          n281 = property on="电机急停" class="Bool (严格)"() -> ("Value"=w374:bool)  [unwired: 2 in, 2 out]
                          n282 = property on="Y(mm)" class="DigNum (严格)"("Value"=w375) -> ()  [unwired: 2 in, 2 out]
                          n283 = case shown="真" w374 {
                            tunnel: w371 -> [_ w380]
                            frame False {
                            }
                            frame True {
                              n284 = call "步进电机命令输入与输出.vi"("输入字符串"="S0/", "串口通信端口"=w380) -> ()  [unwired: 1 out]
                            }
                          }
                          n285 = Subtract(x=w378, y=w375) -> (x-y=w373:dbl)
                          n286 = Absolute Value(x=w373) -> (abs(x)=w372:dbl)
                          n287 = local read "精度"() -> (w376:dbl)
                          n288 = Less?(x=w372, y=w376) -> (x < y?=w377:bool)
                        }
                      }
                      frame True {
                        n289 = flat-sequence {
                          tunnel: [w390] -> _
                          tunnel: [w390] -> w387
                          tunnel: w385 -> [w390]
                          tunnel: [w388] -> w384
                          tunnel: w383 -> [w389]
                          tunnel: w382 -> [w388]
                          frame #0 {
                            n290 = Multiply(x=0.0, y=200.0) -> (x*y=w394:dbl)
                            n291 = Multiply(x=w394, y=w388) -> (x*y=w399:dbl)
                            n292 = Number To Fractional String(number=w399, precision (6)=i16 0 ("精度(6)")) -> (F-format string=w397:string)  [unwired: 2 out]
                            n293 = Concatenate Strings("Y=" ("字符串"), w397, "/" ("字符串")) -> (w392:string)
                            n294 = call "步进电机命令输入与输出.vi"("输入字符串"=w392, "串口通信端口"=w390) -> ()  [unwired: 1 out]
                            n295 = Wait (ms)(milliseconds to wait=w389) -> ()  [unwired: 1 out]
                          }
                        }
                        n296 = while {
                          shift-right: [w401] -> w386
                          shift-left: w387 -> [w401]
                          shift-right: [w400] -> _
                          shift-left: w384 -> [w400]
                          stop <- w407 stop-if-true
                          n297 = property on="电机急停" class="Bool (严格)"() -> ("Value"=w408:bool)  [unwired: 2 in, 2 out]
                          n298 = call "X,Y,Z轴坐标查询.vi"("细分设置"=w400, "查询坐标轴"="Y", "串口通信端口"=w401) -> ("坐标(mm)"=w409:dbl)
                          n299 = case shown="真" w408 {
                            tunnel: w401 -> [_ w412]
                            frame False {
                            }
                            frame True {
                              n300 = call "步进电机命令输入与输出.vi"("输入字符串"="S0/", "串口通信端口"=w412) -> ()  [unwired: 1 out]
                            }
                          }
                          n301 = Multiply(x=w409, y=1.0 ("x")) -> (x*y=w405:dbl)
                          n302 = Subtract(x=w405, y=0.0 ("x")) -> (x-y=w403:dbl)
                          n303 = local read "精度"() -> (w406:dbl)
                          n304 = Absolute Value(x=w403) -> (abs(x)=w402:dbl)
                          n305 = property on="Y(mm)" class="DigNum (严格)"("Value"=w405) -> ()  [unwired: 2 in, 2 out]
                          n306 = Less?(x=w402, y=w406) -> (x < y?=w407:bool)
                        }
                      }
                    }
                    "Y序" <- w268
                  }
                  n307 = property on="已用时（s）" class="DigNum (严格)"("Visible"=TRUE ("可见")) -> ()  [unwired: 2 in, 2 out]
                  n308 = flat-sequence {
                    tunnel: [w193] -> w176
                    tunnel: ["文件保存"] -> w174
                    tunnel: w174 -> [w198]
                    tunnel: [w197] -> w173
                    frame #0 {
                      n309 = Build Path(base path="文件保存", name or relative path="频域谱" ("名称或相对路径")) -> (appended path=w196:path)
                      n310 = Create Folder(path (use dialog)=w196) -> (created path=w193:path)  [unwired: 2 in, 2 out]
                    }
                    frame #1 {
                      n311 = Build Path(base path=w198, name or relative path="时域谱" ("名称或相对路径")) -> (appended path=w199:path)
                      n312 = Create Folder(path (use dialog)=w199) -> (created path=w197:path)  [unwired: 2 in, 2 out]
                    }
                  }
                  n313 = flat-sequence {
                    tunnel: w188 -> [w203]
                    tunnel: [w201] -> _
                    tunnel: [w201] -> w170
                    tunnel: [w203] -> w169
                    tunnel: w168 -> [w201]
                    tunnel: [w204] -> w187
                    tunnel: w170 -> [w204]
                    tunnel: w169 -> [w207]
                    frame #0 {
                      n314 = property on="水平进度条" class="Slide (严格)"("Value"=u8 100 ("水平进度条")) -> ()  [unwired: 2 in, 2 out]
                    }
                    frame #1 {
                      n315 = local read "毫秒计时值"() -> (w206:u32)
                      n316 = Tick Count (ms)() -> (millisecond timer value=w211:u32)
                      n317 = Transpose 2D Array(2D array=w207) -> (transposed array=w208:dbl[][])
                      n318 = Subtract(x=w211, y=w206) -> (x-y=w209:u32)
                      n319 = property on="强度图" class="IntGraph (严格)"("Value"=w208) -> ()  [unwired: 2 in, 2 out]
                      n320 = Multiply(x=w209, y=0.001) -> (x*y=w205:dbl)
                      n321 = property on="已用时（s）" class="DigNum (严格)"("Value"=w205) -> ()  [unwired: 2 in, 2 out]
                      "数组" <- w207
                    }
                  }
                }
                event "逐行扫描": Value Change {
                  n322 = event-data() -> ()  [unwired: 1 in, 6 out]
                  n323 = flat-sequence {
                    tunnel: [w597] -> w510
                    tunnel: [w596] -> w507
                    tunnel: w510 -> [w601]
                    tunnel: [w600] -> w509
                    frame #0 {
                      n324 = local read "文件保存"() -> (w597:path)
                      n325 = Build Path(base path=w597, name or relative path="频域谱" ("名称或相对路径")) -> (appended path=w599:path)
                      n326 = Create Folder(path (use dialog)=w599) -> (created path=w596:path)  [unwired: 2 in, 2 out]
                    }
                    frame #1 {
                      n327 = Build Path(base path=w601, name or relative path="时域谱" ("名称或相对路径")) -> (appended path=w602:path)
                      n328 = Create Folder(path (use dialog)=w602) -> (created path=w600:path)  [unwired: 2 in, 2 out]
                    }
                  }
                  n329 = flat-sequence {
                    tunnel: [w554] -> w505
                    tunnel: w506 -> [w554]
                    frame #0 {
                      # "如果强度图那里出了错，就把这里的行列互换"
                      n330 = property on="Y起点" class="DigNum (严格)"() -> ("Value"=w557:dbl)  [unwired: 2 in, 2 out]
                      n331 = property on="细分设置" class="DigNum (严格)"() -> ("Value"=w555:dbl)  [unwired: 2 in, 2 out]
                      n332 = local read "Xloop"() -> (w561:dbl)
                      n333 = local read "Yloop"() -> (w560:dbl)
                      n334 = Multiply(x=w557, y=200.0) -> (x*y=w565:dbl)
                      n335 = Tick Count (ms)() -> (millisecond timer value=w558:u32)
                      n336 = Multiply(x=w565, y=w555) -> (x*y=w570:dbl)
                      n337 = Initialize Array(0.0 ("元素"), w561, w560) -> (w556:dbl[][])
                      n338 = Number To Fractional String(number=w570, precision (6)=i16 0 ("精度(6)")) -> (F-format string=w568:string)  [unwired: 2 out]
                      n339 = property on="毫秒计时值" class="DigNum (严格)"("Value"=w558) -> ()  [unwired: 2 in, 2 out]
                      n340 = property on="强度图" class="IntGraph (严格)"("Value"=w556) -> ()  [unwired: 2 in, 2 out]
                      n341 = Concatenate Strings("Y=" ("字符串"), w568, "/" ("字符串")) -> (w563:string)
                      n342 = call "步进电机命令输入与输出.vi"("输入字符串"=w563, "串口通信端口"=w554) -> ()  [unwired: 1 out]
                      n343 = property on="等待时间" class="DigNum (严格)"() -> ("Value"=w559:u32)  [unwired: 2 in, 2 out]
                      n344 = property on="已用时（s）" class="DigNum (严格)"("Value"=0.0 ("已用时（s）")) -> ()  [unwired: 2 in, 2 out]
                      n345 = Wait (ms)(milliseconds to wait=w559) -> ()  [unwired: 1 out]
                    }
                  }
                  n346 = property on="水平进度条" class="Slide (严格)"("Visible"=TRUE ("可见")) -> ()  [unwired: 2 in, 2 out]
                  n347 = property on="单行？" class="RadioBtnsControl (严格)"("Visible"=FALSE ("可见")) -> ()  [unwired: 2 in, 2 out]
                  n348 = flat-sequence {
                    tunnel: [w549] -> w504
                    frame #0 {
                      n349 = property on="X终点" class="DigNum (严格)"() -> ("Value"=w538:dbl)  [unwired: 2 in, 2 out]
                      n350 = property on="X起点" class="DigNum (严格)"() -> ("Value"=w537:dbl)  [unwired: 2 in, 2 out]
                      n351 = Subtract(x=w538, y=w537) -> (x-y=w542:dbl)
                      n352 = local read "X:"() -> (w541:dbl)
                      n353 = property on="X扫描范围" class="DigNum (严格)"("Value"=w542) -> ()  [unwired: 2 in, 2 out]
                      n354 = Divide(x=w542, y=w541) -> (x/y=w540:dbl)
                      n355 = Increment(x=w540) -> (x+1=w539:dbl)
                      n356 = property on="Xloop" class="DigNum (严格)"("Value"=w539) -> ()  [unwired: 2 in, 2 out]
                    }
                    frame #1 {
                      n357 = property on="Y终点" class="DigNum (严格)"() -> ("Value"=w544:dbl)  [unwired: 2 in, 2 out]
                      n358 = property on="Y起点" class="DigNum (严格)"() -> ("Value"=w543:dbl)  [unwired: 2 in, 2 out]
                      n359 = Subtract(x=w544, y=w543) -> (x-y=w547:dbl)
                      n360 = local read "Y:"() -> (w546:dbl)
                      n361 = property on="Y扫描范围" class="DigNum (严格)"("Value"=w547) -> ()  [unwired: 2 in, 2 out]
                      n362 = Divide(x=w547, y=w546) -> (x/y=w548:dbl)
                      n363 = Increment(x=w548) -> (x+1=w545:dbl)
                      n364 = property on="Yloop" class="DigNum (严格)"("Value"=w545) -> ()  [unwired: 2 in, 2 out]
                    }
                    frame #2 {
                      n365 = property on="Xloop" class="DigNum (严格)"() -> ("Value"=w552:dbl)  [unwired: 2 in, 2 out]
                      n366 = property on="Yloop" class="DigNum (严格)"() -> ("Value"=w549:dbl)  [unwired: 2 in, 2 out]
                      n367 = Initialize Array(0.0 ("元素"), w552, w549) -> (w551:dbl[][])
                      n368 = property on="强度图" class="IntGraph (严格)"("Value"=w551) -> ()  [unwired: 2 in, 2 out]
                    }
                  }
                  n369 = while {
                    shift-right: [w572] -> w494
                    shift-left: w505 -> [w572]
                    stop <- w577 stop-if-true
                    n370 = call "X,Y,Z轴坐标查询.vi"("细分设置"=8.0, "查询坐标轴"="Y", "串口通信端口"=w572) -> ("坐标(mm)"=w579:dbl)
                    n371 = property on="Y起点" class="DigNum (严格)"() -> ("Value"=w571:dbl)  [unwired: 2 in, 2 out]
                    n372 = property on="电机急停" class="Bool (严格)"() -> ("Value"=w578:bool)  [unwired: 2 in, 2 out]
                    n373 = Multiply(x=w579, y=1.0 ("x")) -> (x*y=w575:dbl)
                    n374 = Subtract(x=w571, y=w575) -> (x-y=w574:dbl)
                    n375 = case shown="真" w578 {
                      tunnel: w572 -> [_ w583]
                      frame False {
                      }
                      frame True {
                        n376 = call "步进电机命令输入与输出.vi"("输入字符串"="S0/", "串口通信端口"=w583) -> ()  [unwired: 1 out]
                      }
                    }
                    n377 = Absolute Value(x=w574) -> (abs(x)=w573:dbl)
                    n378 = local read "精度"() -> (w576:dbl)
                    n379 = property on="Y(mm)" class="DigNum (严格)"("Value"=w575) -> ()  [unwired: 2 in, 2 out]
                    n380 = Less?(x=w573, y=w576) -> (x < y?=w577:bool)
                  }
                  n381 = flat-sequence {
                    tunnel: w494 -> [w514]
                    tunnel: [w514] -> w496
                    tunnel: [w511] -> w495
                    frame #0 {
                      n382 = property on="细分设置" class="DigNum (严格)"() -> ("Value"=w511:dbl)  [unwired: 2 in, 2 out]
                      n383 = Multiply(x=0.0, y=50.0) -> (x*y=w517:dbl)
                      n384 = Multiply(x=w517, y=w511) -> (x*y=w522:dbl)
                      n385 = Number To Fractional String(number=w522, precision (6)=i16 0 ("精度(6)")) -> (F-format string=w520:string)  [unwired: 2 out]
                      n386 = Concatenate Strings("X=" ("字符串"), w520, "/" ("字符串")) -> (w515:string)
                      n387 = call "步进电机命令输入与输出.vi"("输入字符串"=w515, "串口通信端口"=w514) -> ()  [unwired: 1 out]
                      n388 = property on="等待时间" class="DigNum (严格)"() -> ("Value"=w512:u32)  [unwired: 2 in, 2 out]
                      n389 = Wait (ms)(milliseconds to wait=w512) -> ()  [unwired: 1 out]
                    }
                  }
                  n390 = while {
                    shift-right: [w524] -> w493
                    shift-left: w496 -> [w524]
                    shift-right: [w523] -> _
                    shift-left: w495 -> [w523]
                    stop <- w530 stop-if-true
                    n391 = property on="电机急停" class="Bool (严格)"() -> ("Value"=w531:bool)  [unwired: 2 in, 2 out]
                    n392 = call "X,Y,Z轴坐标查询.vi"("细分设置"=w523, "查询坐标轴"="X", "串口通信端口"=w524) -> ("坐标(mm)"=w532:dbl)
                    n393 = case shown="真" w531 {
                      tunnel: w524 -> [_ w535]
                      frame False {
                      }
                      frame True {
                        n394 = call "步进电机命令输入与输出.vi"("输入字符串"="S0/", "串口通信端口"=w535) -> ()  [unwired: 1 out]
                      }
                    }
                    n395 = Multiply(x=w532, y=4.0 ("x")) -> (x*y=w528:dbl)
                    n396 = Subtract(x=0.0, y=w528) -> (x-y=w527:dbl)
                    n397 = Absolute Value(x=w527) -> (abs(x)=w526:dbl)
                    n398 = local read "精度"() -> (w529:dbl)
                    n399 = property on="X（mm）" class="DigNum (严格)"("Value"=w528) -> ()  [unwired: 2 in, 2 out]
                    n400 = Less?(x=w526, y=w529) -> (x < y?=w530:bool)
                  }
                  n401 = for {
                    N: w504 -> [_]
                    shift-right: [w619] -> _
                    shift-left: w507 -> [w619]
                    shift-right: [w618] -> _
                    shift-left: w509 -> [w618]
                    tunnel: [w617] -> w503 mode=indexing
                    shift-right: [w610] -> w502
                    shift-left: w493 -> [w612]
                    i -> [w605]
                    # "实时成像出问题调这里"
                    n402 = local read "Yloop"() -> (w607:dbl)
                    n403 = property on="Y序" class="DigNum (严格)"("Value"=w605) -> ()  [unwired: 2 in, 2 out]
                    n404 = Multiply(x=w607, y=0.01) -> (x*y=w606:dbl)
                    n405 = Divide(x=w605, y=w606) -> (x/y=w608:dbl)
                    n406 = property on="水平进度条" class="Slide (严格)"("Value"=w608) -> ()  [unwired: 2 in, 2 out]
                    n407 = case shown="\"单行\", 默认" "单行？" {
                      tunnel: w619 -> [w630 w705]
                      tunnel: w618 -> [w629 w706]
                      tunnel: [w628 w702] -> w617
                      tunnel: [w624 w700] -> w615
                      tunnel: w612 -> [w623 w704]
                      frame "单行", Default {
                        n408 = flat-sequence {
                          tunnel: [w664] -> w633
                          tunnel: [w662] -> w632
                          tunnel: [w665] -> w628
                          tunnel: [w663] -> w631
                          tunnel: w623 -> [w661]
                          tunnel: [w695] -> w625
                          tunnel: w629 -> [w679]
                          tunnel: w630 -> [w678]
                          tunnel: w633 -> [w691]
                          tunnel: w632 -> [w695]
                          tunnel: w631 -> [w683]
                          frame #0 {
                            n409 = local read "精度"() -> (w673:dbl)
                            n410 = property on="细分设置" class="DigNum (严格)"() -> ("Value"=w672:dbl)  [unwired: 2 in, 2 out]
                            n411 = property on="X终点" class="DigNum (严格)"() -> ("Value"=w676:dbl)  [unwired: 2 in, 2 out]
                            n412 = property on="X起点" class="DigNum (严格)"() -> ("Value"=w660:dbl)  [unwired: 2 in, 2 out]
                            n413 = local read "pulDDR2Length"() -> (w668:u32)
                            n414 = local read "M_Length"() -> (w670:i32)
                            n415 = property on="hDevice" class="DigNum (严格)"() -> ("Value"=w669:i32)  [unwired: 2 in, 2 out]
                            n416 = property on="N_Length" class="DigNum (严格)"() -> ("Value"=w671:i32)  [unwired: 2 in, 2 out]
                            n417 = property on="等待时间" class="DigNum (严格)"() -> ("Value"=w674:u32)  [unwired: 2 in, 2 out]
                            n418 = property on="电机急停" class="Bool (严格)"() -> ("Value"=w675:bool)  [unwired: 2 in, 2 out]
                            n419 = call "X轴连续扫描（1.0）.vi"("VISA I"=w661, "X0"=w660, "X"=w676, "精度"=w673, "细分设置"=w672, "等待时间(ms)"=w674, "pulDDR2Length"=w668, "电机急停"=w675, "hDevice"=w669, "M-length"=w670, "N-length"=w671) -> ("VISA O"=w662:refnum<visa-resource-name>, "hDevice out"=w667:i32, "X"=w666:dbl, "强度图行"=w665:dbl[], "时域谱页"=w664:dbl[][], "幅频谱页"=w663:dbl[][])  [unwired: 3 in]
                            n420 = property on="hDevice 2" class="DigNum (严格)"("Value"=w667) -> ()  [unwired: 2 in, 2 out]
                            n421 = property on="X（mm）" class="DigNum (严格)"("Value"=w666) -> ()  [unwired: 2 in, 2 out]
                          }
                          frame #1 {
                            n422 = property on="Y序" class="DigNum (严格)"() -> ("Value"=w677:i32)  [unwired: 2 in, 2 out]
                            n423 = Increment(x=w677) -> (x+1=w680:i32)
                            n424 = Number To Decimal String(number=w680) -> (decimal integer string=w689:string)  [unwired: 1 in]
                            n425 = Number To Decimal String(number=w680) -> (decimal integer string=w688:string)  [unwired: 1 in]
                            n426 = Concatenate Strings("T" ("字符串"), w689, ".txt" ("字符串")) -> (w692:string)
                            n427 = Concatenate Strings("F" ("字符串"), w688, ".txt" ("字符串")) -> (w686:string)
                            n428 = Build Path(base path=w679, name or relative path=w692) -> (appended path=w694:path)
                            n429 = call-poly <vilib>:"Write Delimited Spreadsheet.vi"("file path (dialog if empty)"=w694, "2D data"=w691, "transpose? (no:F)"=FALSE) -> ()  [unwired: 11 in, 2 out]
                            n430 = Build Path(base path=w678, name or relative path=w686) -> (appended path=w684:path)
                            n431 = call-poly <vilib>:"Write Delimited Spreadsheet.vi"("file path (dialog if empty)"=w684, "2D data"=w683, "transpose? (no:F)"=FALSE) -> ()  [unwired: 11 in, 2 out]
                          }
                        }
                        n432 = flat-sequence {
                          tunnel: w625 -> [w637]
                          tunnel: [w637] -> w626
                          tunnel: [w636] -> w627
                          frame #0 {
                            n433 = property on="细分设置" class="DigNum (严格)"() -> ("Value"=w636:dbl)  [unwired: 2 in, 2 out]
                            n434 = Multiply(x=0.0, y=50.0) -> (x*y=w640:dbl)
                            n435 = Multiply(x=w640, y=w636) -> (x*y=w645:dbl)
                            n436 = local read "等待时间"() -> (w635:u32)
                            n437 = Number To Fractional String(number=w645, precision (6)=i16 0 ("精度(6)")) -> (F-format string=w643:string)  [unwired: 2 out]
                            n438 = Concatenate Strings("X=" ("字符串"), w643, "/" ("字符串")) -> (w638:string)
                            n439 = Wait (ms)(milliseconds to wait=w635) -> ()  [unwired: 1 out]
                            n440 = call "步进电机命令输入与输出.vi"("输入字符串"=w638, "串口通信端口"=w637) -> ()  [unwired: 1 out]
                          }
                        }
                        n441 = while {
                          shift-right: [w649] -> w624
                          shift-left: w626 -> [w649]
                          shift-right: [w647] -> _
                          shift-left: w627 -> [w647]
                          stop <- w653 stop-if-true
                          n442 = property on="电机急停" class="Bool (严格)"() -> ("Value"=w654:bool)  [unwired: 2 in, 2 out]
                          n443 = case shown="真" w654 {
                            tunnel: w649 -> [_ w658]
                            frame False {
                            }
                            frame True {
                              n444 = call "步进电机命令输入与输出.vi"("输入字符串"="S0/", "串口通信端口"=w658) -> ()  [unwired: 1 out]
                            }
                          }
                          n445 = call "X,Y,Z轴坐标查询.vi"("细分设置"=w647, "查询坐标轴"="X", "串口通信端口"=w649) -> ("坐标(mm)"=w655:dbl)
                          n446 = Multiply(x=w655, y=4.0 ("x")) -> (x*y=w651:dbl)
                          n447 = Subtract(x=0.0, y=w651) -> (x-y=w650:dbl)
                          n448 = local read "精度"() -> (w652:dbl)
                          n449 = Absolute Value(x=w650) -> (abs(x)=w648:dbl)
                          n450 = property on="X（mm）" class="DigNum (严格)"("Value"=w651) -> ()  [unwired: 2 in, 2 out]
                          n451 = Less?(x=w648, y=w652) -> (x < y?=w653:bool)
                        }
                      }
                      frame "双行" {
                        n452 = flat-sequence {
                          tunnel: [w747] -> w709
                          tunnel: [w745] -> w708
                          tunnel: [w748] -> w702
                          tunnel: [w746] -> w707
                          tunnel: w704 -> [w744]
                          tunnel: [w741] -> w703
                          tunnel: [w801] -> w701
                          tunnel: w706 -> [w785]
                          tunnel: w705 -> [w784]
                          tunnel: w709 -> [w797]
                          tunnel: w708 -> [w801]
                          tunnel: w707 -> [w789]
                          tunnel: w703 -> [w783]
                          tunnel: [w783] -> w696
                          frame #0 {
                            n453 = property on="Y序" class="DigNum (严格)"() -> ("Value"=w741:i32)  [unwired: 2 in, 2 out]
                            n454 = Power Of X(1:-1.0 ("x"), 2:w741) -> (0:w742:dbl)
                            n455 = case shown="-1" w742 {
                              tunnel: [w750 w771] -> w748
                              tunnel: [w753 w770] -> w747
                              tunnel: [w752 w769] -> w746
                              tunnel: [w751 w768] -> w745
                              tunnel: w744 -> [w749 w767]
                              frame -1 {
                                n456 = local read "精度"() -> (w762:dbl)
                                n457 = property on="细分设置" class="DigNum (严格)"() -> ("Value"=w761:dbl)  [unwired: 2 in, 2 out]
                                n458 = property on="X终点" class="DigNum (严格)"() -> ("Value"=w765:dbl)  [unwired: 2 in, 2 out]
                                n459 = property on="X起点" class="DigNum (严格)"() -> ("Value"=w754:dbl)  [unwired: 2 in, 2 out]
                                n460 = local read "pulDDR2Length"() -> (w757:u32)
                                n461 = local read "M_Length"() -> (w759:i32)
                                n462 = property on="hDevice" class="DigNum (严格)"() -> ("Value"=w758:i32)  [unwired: 2 in, 2 out]
                                n463 = property on="N_Length" class="DigNum (严格)"() -> ("Value"=w760:i32)  [unwired: 2 in, 2 out]
                                n464 = property on="等待时间" class="DigNum (严格)"() -> ("Value"=w763:u32)  [unwired: 2 in, 2 out]
                                n465 = property on="电机急停" class="Bool (严格)"() -> ("Value"=w764:bool)  [unwired: 2 in, 2 out]
                                n466 = call "X轴回程连续扫描（1.0）.vi"("VISA I"=w749, "X0"=w754, "X"=w765, "精度"=w762, "细分设置"=w761, "等待时间(ms)"=w763, "pulDDR2Length"=w757, "电机急停"=w764, "hDevice"=w758, "M-length"=w759, "N-length"=w760) -> ("VISA O"=w751:refnum<visa-resource-name>, "hDevice out"=w756:i32, "X"=w755:dbl, "强度图行"=w750:dbl[], "时域谱页"=w753:dbl[][], "幅频谱页"=w752:dbl[][])  [unwired: 3 in]
                                n467 = property on="hDevice 2" class="DigNum (严格)"("Value"=w756) -> ()  [unwired: 2 in, 2 out]
                                n468 = property on="X（mm）" class="DigNum (严格)"("Value"=w755) -> ()  [unwired: 2 in, 2 out]
                              }
                              frame 1, Default {
                                n469 = local read "精度"() -> (w779:dbl)
                                n470 = property on="细分设置" class="DigNum (严格)"() -> ("Value"=w778:dbl)  [unwired: 2 in, 2 out]
                                n471 = property on="X终点" class="DigNum (严格)"() -> ("Value"=w782:dbl)  [unwired: 2 in, 2 out]
                                n472 = property on="X起点" class="DigNum (严格)"() -> ("Value"=w766:dbl)  [unwired: 2 in, 2 out]
                                n473 = local read "pulDDR2Length"() -> (w774:u32)
                                n474 = local read "M_Length"() -> (w776:i32)
                                n475 = property on="hDevice" class="DigNum (严格)"() -> ("Value"=w775:i32)  [unwired: 2 in, 2 out]
                                n476 = property on="N_Length" class="DigNum (严格)"() -> ("Value"=w777:i32)  [unwired: 2 in, 2 out]
                                n477 = property on="等待时间" class="DigNum (严格)"() -> ("Value"=w780:u32)  [unwired: 2 in, 2 out]
                                n478 = property on="电机急停" class="Bool (严格)"() -> ("Value"=w781:bool)  [unwired: 2 in, 2 out]
                                n479 = call "X轴连续扫描（1.0）.vi"("VISA I"=w767, "X0"=w766, "X"=w782, "精度"=w779, "细分设置"=w778, "等待时间(ms)"=w780, "pulDDR2Length"=w774, "电机急停"=w781, "hDevice"=w775, "M-length"=w776, "N-length"=w777) -> ("VISA O"=w768:refnum<visa-resource-name>, "hDevice out"=w773:i32, "X"=w772:dbl, "强度图行"=w771:dbl[], "时域谱页"=w770:dbl[][], "幅频谱页"=w769:dbl[][])  [unwired: 3 in]
                                n480 = property on="hDevice 2" class="DigNum (严格)"("Value"=w773) -> ()  [unwired: 2 in, 2 out]
                                n481 = property on="X（mm）" class="DigNum (严格)"("Value"=w772) -> ()  [unwired: 2 in, 2 out]
                              }
                            }
                          }
                          frame #1 {
                            n482 = Increment(x=w783) -> (x+1=w786:i32)
                            n483 = Number To Decimal String(number=w786) -> (decimal integer string=w795:string)  [unwired: 1 in]
                            n484 = Number To Decimal String(number=w786) -> (decimal integer string=w794:string)  [unwired: 1 in]
                            n485 = Concatenate Strings("T" ("字符串"), w795, ".txt" ("字符串")) -> (w798:string)
                            n486 = Concatenate Strings("F" ("字符串"), w794, ".txt" ("字符串")) -> (w792:string)
                            n487 = Build Path(base path=w785, name or relative path=w798) -> (appended path=w800:path)
                            n488 = call-poly <vilib>:"Write Delimited Spreadsheet.vi"("file path (dialog if empty)"=w800, "2D data"=w797, "transpose? (no:F)"=FALSE) -> ()  [unwired: 11 in, 2 out]
                            n489 = Build Path(base path=w784, name or relative path=w792) -> (appended path=w790:path)
                            n490 = call-poly <vilib>:"Write Delimited Spreadsheet.vi"("file path (dialog if empty)"=w790, "2D data"=w789, "transpose? (no:F)"=FALSE) -> ()  [unwired: 11 in, 2 out]
                          }
                        }
                        n491 = property on="Yloop" class="DigNum (严格)"() -> ("Value"=w699:dbl)  [unwired: 2 in, 2 out]
                        n492 = Decrement(x=w699) -> (x-1=w698:dbl)
                        n493 = Equal?(x=w696, y=w698) -> (x = y?=w697:bool)
                        n494 = case shown="真" w697 {
                          tunnel: w701 -> [w710 w711]
                          tunnel: [w710 w712] -> w700
                          frame False {
                          }
                          frame True {
                            n495 = flat-sequence {
                              tunnel: w711 -> [w718]
                              tunnel: [w718] -> w713
                              tunnel: [w717] -> w714
                              frame #0 {
                                n496 = property on="细分设置" class="DigNum (严格)"() -> ("Value"=w717:dbl)  [unwired: 2 in, 2 out]
                                n497 = Multiply(x=0.0, y=50.0) -> (x*y=w721:dbl)
                                n498 = Multiply(x=w721, y=w717) -> (x*y=w726:dbl)
                                n499 = local read "等待时间"() -> (w716:u32)
                                n500 = Number To Fractional String(number=w726, precision (6)=i16 0 ("精度(6)")) -> (F-format string=w724:string)  [unwired: 2 out]
                                n501 = Concatenate Strings("X=" ("字符串"), w724, "/" ("字符串")) -> (w719:string)
                                n502 = Wait (ms)(milliseconds to wait=w716) -> ()  [unwired: 1 out]
                                n503 = call "步进电机命令输入与输出.vi"("输入字符串"=w719, "串口通信端口"=w718) -> ()  [unwired: 1 out]
                              }
                            }
                            n504 = while {
                              shift-right: [w730] -> w712
                              shift-left: w713 -> [w730]
                              shift-right: [w728] -> _
                              shift-left: w714 -> [w728]
                              stop <- w734 stop-if-true
                              n505 = property on="电机急停" class="Bool (严格)"() -> ("Value"=w735:bool)  [unwired: 2 in, 2 out]
                              n506 = case shown="真" w735 {
                                tunnel: w730 -> [_ w739]
                                frame False {
                                }
                                frame True {
                                n507 = call "步进电机命令输入与输出.vi"("输入字符串"="S0/", "串口通信端口"=w739) -> ()  [unwired: 1 out]
                                }
                              }
                              n508 = call "X,Y,Z轴坐标查询.vi"("细分设置"=w728, "查询坐标轴"="X", "串口通信端口"=w730) -> ("坐标(mm)"=w736:dbl)
                              n509 = Multiply(x=w736, y=4.0 ("x")) -> (x*y=w732:dbl)
                              n510 = Subtract(x=0.0, y=w732) -> (x-y=w731:dbl)
                              n511 = local read "精度"() -> (w733:dbl)
                              n512 = Absolute Value(x=w731) -> (abs(x)=w729:dbl)
                              n513 = property on="X（mm）" class="DigNum (严格)"("Value"=w732) -> ()  [unwired: 2 in, 2 out]
                              n514 = Less?(x=w729, y=w733) -> (x < y?=w734:bool)
                            }
                          }
                        }
                      }
                    }
                    n515 = property on="强度图" class="IntGraph (严格)"() -> ("Value"=w622:dbl[][])  [unwired: 2 in, 2 out]
                    n516 = property on="Yloop" class="DigNum (严格)"() -> ("Value"=w613:dbl)  [unwired: 2 in, 2 out]
                    n517 = property on="Y序" class="DigNum (严格)"() -> ("Value"=w616:i32)  [unwired: 2 in, 2 out]
                    n518 = Replace Array Subset(array=w622, new element=w617, index (col)=w616) -> (w621:dbl[][])  [unwired: 1 in]
                    n519 = property on="强度图" class="IntGraph (严格)"("Value"=w621) -> ()  [unwired: 2 in, 2 out]
                    n520 = Decrement(x=w613) -> (x-1=w614:dbl)
                    n521 = Equal?(x=w616, y=w614) -> (x = y?=w620:bool)
                    n522 = case shown="真" w620 {
                      tunnel: w615 -> [w811 w841]
                      tunnel: [w809 w842] -> w611
                      frame False {
                        n523 = flat-sequence {
                          tunnel: w811 -> [w815]
                          tunnel: [w815] -> w810
                          tunnel: [w812] -> w808
                          frame #0 {
                            n524 = property on="细分设置" class="DigNum (严格)"() -> ("Value"=w812:dbl)  [unwired: 2 in, 2 out]
                            n525 = call "X,Y,Z轴坐标查询.vi"("细分设置"=w812, "查询坐标轴"="Y", "串口通信端口"=w815) -> ("坐标(mm)"=w816:dbl)
                            n526 = property on="Y:" class="DigNum (严格)"() -> ("Value"=w814:dbl)  [unwired: 2 in, 2 out]
                            n527 = Add(x=w816, y=w814) -> (x+y=w818:dbl)
                            "x+y 3" <- w818
                            n528 = Multiply(x=w818, y=200.0) -> (x*y=w822:dbl)
                            n529 = Multiply(x=w822, y=8.0 ("细分设置")) -> (x*y=w827:dbl)
                            n530 = Number To Fractional String(number=w827, precision (6)=i16 0 ("精度(6)")) -> (F-format string=w825:string)  [unwired: 2 out]
                            n531 = Concatenate Strings("Y=" ("字符串"), w825, "/" ("字符串")) -> (w820:string)
                            n532 = call "步进电机命令输入与输出.vi"("输入字符串"=w820, "串口通信端口"=w815) -> ()  [unwired: 1 out]
                            n533 = property on="等待时间" class="DigNum (严格)"() -> ("Value"=w813:u32)  [unwired: 2 in, 2 out]
                            n534 = Wait (ms)(milliseconds to wait=w813) -> ()  [unwired: 1 out]
                          }
                        }
                        n535 = while {
                          shift-right: [w830] -> w809
                          shift-left: w810 -> [w830]
                          shift-right: [w829] -> _
                          shift-left: w808 -> [w829]
                          stop <- w836 stop-if-true
                          n536 = call "X,Y,Z轴坐标查询.vi"("细分设置"=w829, "查询坐标轴"="Y", "串口通信端口"=w830) -> ("坐标(mm)"=w834:dbl)
                          n537 = property on="x+y 3" class="DigNum (严格)"() -> ("Value"=w828:dbl)  [unwired: 2 in, 2 out]
                          n538 = property on="电机急停" class="Bool (严格)"() -> ("Value"=w833:bool)  [unwired: 2 in, 2 out]
                          n539 = property on="Y(mm)" class="DigNum (严格)"("Value"=w834) -> ()  [unwired: 2 in, 2 out]
                          n540 = case shown="真" w833 {
                            tunnel: w830 -> [_ w838]
                            frame False {
                            }
                            frame True {
                              n541 = call "步进电机命令输入与输出.vi"("输入字符串"="S0/", "串口通信端口"=w838) -> ()  [unwired: 1 out]
                            }
                          }
                          n542 = Subtract(x=w828, y=w834) -> (x-y=w832:dbl)
                          n543 = Absolute Value(x=w832) -> (abs(x)=w831:dbl)
                          n544 = local read "精度"() -> (w835:dbl)
                          n545 = Less?(x=w831, y=w835) -> (x < y?=w836:bool)
                        }
                      }
                      frame True {
                        n546 = flat-sequence {
                          tunnel: [w846] -> _
                          tunnel: [w846] -> w843
                          tunnel: w841 -> [w846]
                          tunnel: [w844] -> w840
                          frame #0 {
                            n547 = property on="细分设置" class="DigNum (严格)"() -> ("Value"=w844:dbl)  [unwired: 2 in, 2 out]
                            n548 = Multiply(x=0.0, y=200.0) -> (x*y=w850:dbl)
                            n549 = Multiply(x=w850, y=w844) -> (x*y=w855:dbl)
                            n550 = Number To Fractional String(number=w855, precision (6)=i16 0 ("精度(6)")) -> (F-format string=w853:string)  [unwired: 2 out]
                            n551 = Concatenate Strings("Y=" ("字符串"), w853, "/" ("字符串")) -> (w848:string)
                            n552 = call "步进电机命令输入与输出.vi"("输入字符串"=w848, "串口通信端口"=w846) -> ()  [unwired: 1 out]
                            n553 = property on="等待时间" class="DigNum (严格)"() -> ("Value"=w845:u32)  [unwired: 2 in, 2 out]
                            n554 = Wait (ms)(milliseconds to wait=w845) -> ()  [unwired: 1 out]
                          }
                        }
                        n555 = while {
                          shift-right: [w857] -> w842
                          shift-left: w843 -> [w857]
                          shift-right: [w856] -> _
                          shift-left: w840 -> [w856]
                          stop <- w863 stop-if-true
                          n556 = property on="电机急停" class="Bool (严格)"() -> ("Value"=w864:bool)  [unwired: 2 in, 2 out]
                          n557 = call "X,Y,Z轴坐标查询.vi"("细分设置"=w856, "查询坐标轴"="Y", "串口通信端口"=w857) -> ("坐标(mm)"=w865:dbl)
                          n558 = case shown="真" w864 {
                            tunnel: w857 -> [_ w868]
                            frame False {
                            }
                            frame True {
                              n559 = call "步进电机命令输入与输出.vi"("输入字符串"="S0/", "串口通信端口"=w868) -> ()  [unwired: 1 out]
                            }
                          }
                          n560 = Multiply(x=w865, y=1.0 ("x")) -> (x*y=w861:dbl)
                          n561 = Subtract(x=w861, y=0.0 ("x")) -> (x-y=w859:dbl)
                          n562 = local read "精度"() -> (w862:dbl)
                          n563 = Absolute Value(x=w859) -> (abs(x)=w858:dbl)
                          n564 = property on="Y(mm)" class="DigNum (严格)"("Value"=w861) -> ()  [unwired: 2 in, 2 out]
                          n565 = Less?(x=w858, y=w862) -> (x < y?=w863:bool)
                        }
                      }
                    }
                    n566 = flat-sequence {
                      tunnel: w611 -> [w802]
                      tunnel: [w802] -> w610
                      frame #0 {
                        n567 = local read "毫秒计时值"() -> (w803:u32)
                        n568 = Tick Count (ms)() -> (millisecond timer value=w806:u32)
                        n569 = Subtract(x=w806, y=w803) -> (x-y=w804:u32)
                        n570 = Multiply(x=w804, y=0.001) -> (x*y=w807:dbl)
                        n571 = property on="已用时（s）" class="DigNum (严格)"("Value"=w807) -> ()  [unwired: 2 in, 2 out]
                      }
                    }
                  }
                  n572 = property on="已用时（s）" class="DigNum (严格)"("Visible"=TRUE ("可见")) -> ()  [unwired: 2 in, 2 out]
                  n573 = flat-sequence {
                    tunnel: w503 -> [w586]
                    tunnel: w502 -> [w587]
                    tunnel: [w587] -> w499
                    tunnel: [w586] -> w498
                    tunnel: [w589] -> w508
                    tunnel: w499 -> [w589]
                    tunnel: w498 -> [w590]
                    frame #0 {
                      n574 = property on="水平进度条" class="Slide (严格)"("Value"=u8 100 ("水平进度条")) -> ()  [unwired: 2 in, 2 out]
                    }
                    frame #1 {
                      n575 = local read "毫秒计时值"() -> (w594:u32)
                      n576 = property on="数组" class="Arr (严格)"("Value"=w590) -> ()  [unwired: 2 in, 2 out]
                      n577 = Transpose 2D Array(2D array=w590) -> (transposed array=w591:dbl[][])
                      n578 = Tick Count (ms)() -> (millisecond timer value=w595:u32)
                      n579 = property on="强度图" class="IntGraph (严格)"("Value"=w591) -> ()  [unwired: 2 in, 2 out]
                      n580 = Subtract(x=w595, y=w594) -> (x-y=w592:u32)
                      n581 = Multiply(x=w592, y=0.001) -> (x*y=w588:dbl)
                      n582 = property on="已用时（s）" class="DigNum (严格)"("Value"=w588) -> ()  [unwired: 2 in, 2 out]
                    }
                  }
                }
                event "分层图查看": Value Change {
                  n583 = event-data() -> ()  [unwired: 1 in, 6 out]
                  n584 = call "分层图显示1.2.1（导入色码表）.vi"("IN"=w871) -> ("OUT"=w870:string)  [unwired: 10 in]
                }
              }
            }
          }
        }
        n585 = dll-call lib="PTH2]abs CUsersH301Desktopart闭环扫描程序采集卡控制INFamd64\nPCI8502_32" fn="PCI8502_ReleaseDeviceAD" label="ReleaseDeviceAD"("hDevice"="hDevice 2") -> ("hDevice"=w20:i32)  [unwired: 4 in, 2 out]
        n586 = VISA Close(VISA resource name=w18) -> (error out=→"错误输出":errorcluster)  [unwired: 1 in]
        n587 = dll-call lib="PTH2]abs CUsersH301Desktopart闭环扫描程序采集卡控制INFamd64\nPCI8502_32" fn="PCI8502_ReleaseDevice" label="ReleaseDevice"("hDevice"=w20) -> ()  [unwired: 5 in, 2 out]
        "M_Length" <- w24
      }
    }
  }
  n588 = property on="高级设置" class="Bool"("Visible"=FALSE ("可见")) -> ()  [unwired: 2 in, 2 out]
  n589 = property on="定位模式" class="Bool"("Visible"=FALSE ("可见")) -> ()  [unwired: 2 in, 2 out]
  n590 = property on="已用时（s）" class="DigNum (严格)"("Visible"=FALSE ("可见")) -> ()  [unwired: 2 in, 2 out]
